vi "Main.vi"() -> ()   [LabVIEW 2010]
uses:
  <vilib>/Utility/config.llb/Read Key (Path).vi
  <vilib>/Utility/config.llb/Write Key (Path).vi
  DLL-s/MakeFullImmitationStepDLL/Release/MakeFullImmitationStepDLL.dll
  <vilib>/Utility/config.llb/NI_LVConfig.lvlib
panel:
  out "toChanger":T1(array[cluster])
  out "subpanel VI ref":refnum<vi>
  out "VP 2 GUI Msg Cluster Array":cluster{"Names":string[], "Codes":i32[]}
  out "selected path":path
  out "End Number":i32
  out "Project":string
  out "VP input vars":T2
  out "VP output vars":T3
  out "VM input vars":T2
  out "VM2SCM Msg Cluster Array":cluster{"Names":string[], "Codes":i32[]}
  out "VM INP from SCM Msg Cluster Array":cluster{"Names":string[], "Codes":i32[]}
  out "SCM2CA Msg Cluster Array":cluster{"Names":string[], "Codes":i32[]}
  out "SCM-SCM2VP Msg Cluster Array":cluster{"Names":string[], "Codes":i32[]}
  out "SCM2VM Msg Cluster Array":cluster{"Names":string[], "Codes":i32[]}
  out "VM2GUI Msg Cluster Array":cluster{"Names":string[], "Codes":i32[]}
  out "SCM STATES":string[][](array[string])
  out "SCM PROCESSES":string[](array[string])=["Инициализация", "ОстановВсехПроцессовИстартПроцИнициализация", "КонтрольДостоверности", "КонтрольДостоверностиОткрытияЗатвораВакуумного", "КонтрольДостоверностиОткрЗатВакуумного", "КонтрольДостоверностиЗакрЗатВакуумного", "КонтрольДостоверностиСостоянияСапуна", "КонтрольДостоверностиСостоянияУстройстваПлавПуска", "КонтрольДостоверностиСостоянияПитанияВакуумногоНасоса", "КонтрольДостоверностиСостоянияПитанияВентилятора", "КонтрольДостоверностиСостоянияПитанияРегТемпературы", "КонтрольДостоверностиСостоянияПитанияРегУровня", "КонтрольДостоверностиУровняВодыМинимум", "КонтрольДостоверностиУровняВодыМаксимум", "КонтрольДостоверностиСостоянияПитанияНасОхлаждения", "ЧтениеФактПараметров_с_Датчиков", "РЕГУЛЯТОР_ТРАФИКА", "ЧтениеКольцевогоБуфера", "ОбработкаКомандИзмененияНП_от_ГУИ", "ОбработкаКомандУправления_от_ГУИ", "КонтрольИзменения_ФП_P_ВбакеКомпрессора", "КонтрольИзменения_ФП_P_Впатрубке", "КонтрольИзменения_ФП_T_Врубашке", "КонтрольИзменения_ФП_T_Вбаке", "КонтрольИзменения_ФП_P_ВтрубеСидер", "КонтрольВеличиныОткачкиВауумнойТрубыСидеростата", "КонтрольГотовностиВакуума_в_Вакуумной_Трубе", "КонтрольУровняВодыБакаОхлаждения", "КонтрольТемпературыВодыБакаОхлаждения", "КонтрольТемпературыРубашкиОхлаждения", "КонтрольДавленияВбакеКомпрессора", "ВКЛ_ПИТ_ВЕНТИЛЯТОР", "ВЫК_ПИТ_ВЕНТИЛЯТОР", "КонтрольСостоянияПитанияВентилятора", "КонтрольСпонтанногоВыключенияВентилятора", "КонтрольСпонтанногоВключенияВентилятора", "КонтрольСостоянияЗатвораВакуумного", "ОТКР_ЗАТВОР_ВАК", "ЗАКР_ЗАТВОР_ВАК", "КонтрольСпонтанногоЗакрытияЗатвораВакуумного", "КонтрольСпонтанногоОткрытияЗатвораВакуумного", "ОТКР_САПУН", "ЗАКР_САПУН", "КонтрольСостоянияПитанияСапуна", "КонтрольСпонтанногоЗакрытияСапуна", "КонтрольСпонтанногоОткрытияСапуна", "ВКЛ_ПИТ_ВАК_НАСОСА", "ВЫК_ПИТ_ВАК_НАСОСА", "КонтрольСостоянияПитанияВакуумногоНасоса", "КонтрольСпонтанногоВыключенияВакНасоса", "КонтрольСпонтанногоВключенияВакНасоса", "ВКЛ_ПИТ_РЕГ_Т", "ВЫК_ПИТ_РЕГ_Т", "КонтрольСостоянияПитанияРЕГ_Т", "КонтрольСпонтанногоВыключенияРЕГ_Т", "КонтрольСпонтанногоВключенияРЕГ_Т", "ВКЛ_ПИТ_РЕГ_УР", "ВЫК_ПИТ_РЕГ_УР", "КонтрольСостоянияПитанияРЕГ_УР", "КонтрольСпонтанногоВыключенияРЕГ_УР", "КонтрольСпонтанногоВключенияРЕГ_УР", "ВКЛ_ПИТ_НАС_ОХЛ", "ВЫК_ПИТ_НАС_ОХЛ", "КонтрольСостоянияПитанияНАС_ОХЛ", "КонтрольСпонтанногоВыключенияНасосаОхлаждения", "КонтрольСпонтанногоВключенияНасосаОхлаждения", "ВКЛ_УСТР_ПЛАВ_ПУСКА", "ВЫК_УСТР_ПЛАВ_ПУСКА", "КонтрольСостоянияПитанияПЛАВ_ПУСКА", "КонтрольСпонтанногоВыключенияПлавнПуска", "КонтрольСпонтанногоВключенияПлавнПуска", "ВКЛ_ВАКУУМИРОВАНИЕ_ТРУБЫ", "ВЫК_ВАКУУМИРОВАНИЕ_ТРУБЫ", "ВКЛ_ВАКУУМНУЮ_ПОДСИСТЕМУ", "ВЫК_ВАКУУМНУЮ_ПОДСИСТЕМУ"]
  out "VM STATES":string[][](array[string])
  out "VM PROCESSES":string[](array[string])=["Инициализация", "ОстановВсехПроцессовИстартПроцИнициализация", "КонтрольДостоверности", "КонтрольДостоверностиОткрытияЗатвораВакуумного", "КонтрольДостоверностиОткрЗатВакуумного", "КонтрольДостоверностиЗакрЗатВакуумного", "КонтрольДостоверностиСостоянияСапуна", "КонтрольДостоверностиСостоянияУстройстваПлавПуска", "КонтрольДостоверностиСостоянияПитанияВакуумногоНасоса", "КонтрольДостоверностиСостоянияПитанияВентилятора", "КонтрольДостоверностиСостоянияПитанияРегТемпературы", "КонтрольДостоверностиСостоянияПитанияРегУровня", "КонтрольДостоверностиУровняВодыМинимум", "КонтрольДостоверностиУровняВодыМаксимум", "КонтрольДостоверностиСостоянияПитанияНасОхлаждения", "ЧтениеФактПараметров_с_Датчиков", "РЕГУЛЯТОР_ТРАФИКА", "ЧтениеКольцевогоБуфера", "ОбработкаКомандИзмененияНП_от_ГУИ", "ОбработкаКомандУправления_от_ГУИ", "КонтрольИзменения_ФП_P_ВбакеКомпрессора", "КонтрольИзменения_ФП_P_Впатрубке", "КонтрольИзменения_ФП_T_Врубашке", "КонтрольИзменения_ФП_T_Вбаке", "КонтрольИзменения_ФП_P_ВтрубеСидер", "КонтрольВеличиныОткачкиВауумнойТрубыСидеростата", "КонтрольГотовностиВакуума_в_Вакуумной_Трубе", "КонтрольУровняВодыБакаОхлаждения", "КонтрольТемпературыВодыБакаОхлаждения", "КонтрольТемпературыРубашкиОхлаждения", "КонтрольДавленияВбакеКомпрессора", "ВКЛ_ПИТ_ВЕНТИЛЯТОР", "ВЫК_ПИТ_ВЕНТИЛЯТОР", "КонтрольСостоянияПитанияВентилятора", "КонтрольСпонтанногоВыключенияВентилятора", "КонтрольСпонтанногоВключенияВентилятора", "КонтрольСостоянияЗатвораВакуумного", "ОТКР_ЗАТВОР_ВАК", "ЗАКР_ЗАТВОР_ВАК", "КонтрольСпонтанногоЗакрытияЗатвораВакуумного", "КонтрольСпонтанногоОткрытияЗатвораВакуумного", "ОТКР_САПУН", "ЗАКР_САПУН", "КонтрольСостоянияПитанияСапуна", "КонтрольСпонтанногоЗакрытияСапуна", "КонтрольСпонтанногоОткрытияСапуна", "ВКЛ_ПИТ_ВАК_НАСОСА", "ВЫК_ПИТ_ВАК_НАСОСА", "КонтрольСостоянияПитанияВакуумногоНасоса", "КонтрольСпонтанногоВыключенияВакНасоса", "КонтрольСпонтанногоВключенияВакНасоса", "ВКЛ_ПИТ_РЕГ_Т", "ВЫК_ПИТ_РЕГ_Т", "КонтрольСостоянияПитанияРЕГ_Т", "КонтрольСпонтанногоВыключенияРЕГ_Т", "КонтрольСпонтанногоВключенияРЕГ_Т", "ВКЛ_ПИТ_РЕГ_УР", "ВЫК_ПИТ_РЕГ_УР", "КонтрольСостоянияПитанияРЕГ_УР", "КонтрольСпонтанногоВыключенияРЕГ_УР", "КонтрольСпонтанногоВключенияРЕГ_УР", "ВКЛ_ПИТ_НАС_ОХЛ", "ВЫК_ПИТ_НАС_ОХЛ", "КонтрольСостоянияПитанияНАС_ОХЛ", "КонтрольСпонтанногоВыключенияНасосаОхлаждения", "КонтрольСпонтанногоВключенияНасосаОхлаждения", "ВКЛ_УСТР_ПЛАВ_ПУСКА", "ВЫК_УСТР_ПЛАВ_ПУСКА", "КонтрольСостоянияПитанияПЛАВ_ПУСКА", "КонтрольСпонтанногоВыключенияПлавнПуска", "КонтрольСпонтанногоВключенияПлавнПуска", "ВКЛ_ВАКУУМИРОВАНИЕ_ТРУБЫ", "ВЫК_ВАКУУМИРОВАНИЕ_ТРУБЫ", "ВКЛ_ВАКУУМНУЮ_ПОДСИСТЕМУ", "ВЫК_ВАКУУМНУЮ_ПОДСИСТЕМУ"]
  out "VP STATES":string[][](array[string])
  out "VP PROCESSES":string[](array[string])=["Инициализация", "ОстановВсехПроцессовИстартПроцИнициализация", "КонтрольДостоверности", "КонтрольДостоверностиОткрытияЗатвораВакуумного", "КонтрольДостоверностиОткрЗатВакуумного", "КонтрольДостоверностиЗакрЗатВакуумного", "КонтрольДостоверностиСостоянияСапуна", "КонтрольДостоверностиСостоянияУстройстваПлавПуска", "КонтрольДостоверностиСостоянияПитанияВакуумногоНасоса", "КонтрольДостоверностиСостоянияПитанияВентилятора", "КонтрольДостоверностиСостоянияПитанияРегТемпературы", "КонтрольДостоверностиСостоянияПитанияРегУровня", "КонтрольДостоверностиУровняВодыМинимум", "КонтрольДостоверностиУровняВодыМаксимум", "КонтрольДостоверностиСостоянияПитанияНасОхлаждения", "ЧтениеФактПараметров_с_Датчиков", "РЕГУЛЯТОР_ТРАФИКА", "ЧтениеКольцевогоБуфера", "ОбработкаКомандИзмененияНП_от_ГУИ", "ОбработкаКомандУправления_от_ГУИ", "КонтрольИзменения_ФП_P_ВбакеКомпрессора", "КонтрольИзменения_ФП_P_Впатрубке", "КонтрольИзменения_ФП_T_Врубашке", "КонтрольИзменения_ФП_T_Вбаке", "КонтрольИзменения_ФП_P_ВтрубеСидер", "КонтрольВеличиныОткачкиВауумнойТрубыСидеростата", "КонтрольГотовностиВакуума_в_Вакуумной_Трубе", "КонтрольУровняВодыБакаОхлаждения", "КонтрольТемпературыВодыБакаОхлаждения", "КонтрольТемпературыРубашкиОхлаждения", "КонтрольДавленияВбакеКомпрессора", "ВКЛ_ПИТ_ВЕНТИЛЯТОР", "ВЫК_ПИТ_ВЕНТИЛЯТОР", "КонтрольСостоянияПитанияВентилятора", "КонтрольСпонтанногоВыключенияВентилятора", "КонтрольСпонтанногоВключенияВентилятора", "КонтрольСостоянияЗатвораВакуумного", "ОТКР_ЗАТВОР_ВАК", "ЗАКР_ЗАТВОР_ВАК", "КонтрольСпонтанногоЗакрытияЗатвораВакуумного", "КонтрольСпонтанногоОткрытияЗатвораВакуумного", "ОТКР_САПУН", "ЗАКР_САПУН", "КонтрольСостоянияПитанияСапуна", "КонтрольСпонтанногоЗакрытияСапуна", "КонтрольСпонтанногоОткрытияСапуна", "ВКЛ_ПИТ_ВАК_НАСОСА", "ВЫК_ПИТ_ВАК_НАСОСА", "КонтрольСостоянияПитанияВакуумногоНасоса", "КонтрольСпонтанногоВыключенияВакНасоса", "КонтрольСпонтанногоВключенияВакНасоса", "ВКЛ_ПИТ_РЕГ_Т", "ВЫК_ПИТ_РЕГ_Т", "КонтрольСостоянияПитанияРЕГ_Т", "КонтрольСпонтанногоВыключенияРЕГ_Т", "КонтрольСпонтанногоВключенияРЕГ_Т", "ВКЛ_ПИТ_РЕГ_УР", "ВЫК_ПИТ_РЕГ_УР", "КонтрольСостоянияПитанияРЕГ_УР", "КонтрольСпонтанногоВыключенияРЕГ_УР", "КонтрольСпонтанногоВключенияРЕГ_УР", "ВКЛ_ПИТ_НАС_ОХЛ", "ВЫК_ПИТ_НАС_ОХЛ", "КонтрольСостоянияПитанияНАС_ОХЛ", "КонтрольСпонтанногоВыключенияНасосаОхлаждения", "КонтрольСпонтанногоВключенияНасосаОхлаждения", "ВКЛ_УСТР_ПЛАВ_ПУСКА", "ВЫК_УСТР_ПЛАВ_ПУСКА", "КонтрольСостоянияПитанияПЛАВ_ПУСКА", "КонтрольСпонтанногоВыключенияПлавнПуска", "КонтрольСпонтанногоВключенияПлавнПуска", "ВКЛ_ВАКУУМИРОВАНИЕ_ТРУБЫ", "ВЫК_ВАКУУМИРОВАНИЕ_ТРУБЫ", "ВКЛ_ВАКУУМНУЮ_ПОДСИСТЕМУ", "ВЫК_ВАКУУМНУЮ_ПОДСИСТЕМУ"]
  out "VP Cluster":T4
  out "CA output vars":T3
  out "CA input vars":T2
  out "CA2GUI Msg Cluster Array":cluster{"Names":string[], "Codes":i32[]}
  out "COM2CA MSG Cluster Array":cluster{"Names":string[], "Codes":i32[]}
  out "CA STATES":string[][](array[string])
  out "CA PROCESSES":string[](array[string])=["Инициализация", "ОстановВсехПроцессовИстартПроцИнициализация", "КонтрольДостоверности", "КонтрольДостоверностиОткрытияЗатвораВакуумного", "КонтрольДостоверностиОткрЗатВакуумного", "КонтрольДостоверностиЗакрЗатВакуумного", "КонтрольДостоверностиСостоянияСапуна", "КонтрольДостоверностиСостоянияУстройстваПлавПуска", "КонтрольДостоверностиСостоянияПитанияВакуумногоНасоса", "КонтрольДостоверностиСостоянияПитанияВентилятора", "КонтрольДостоверностиСостоянияПитанияРегТемпературы", "КонтрольДостоверностиСостоянияПитанияРегУровня", "КонтрольДостоверностиУровняВодыМинимум", "КонтрольДостоверностиУровняВодыМаксимум", "КонтрольДостоверностиСостоянияПитанияНасОхлаждения", "ЧтениеФактПараметров_с_Датчиков", "РЕГУЛЯТОР_ТРАФИКА", "ЧтениеКольцевогоБуфера", "ОбработкаКомандИзмененияНП_от_ГУИ", "ОбработкаКомандУправления_от_ГУИ", "КонтрольИзменения_ФП_P_ВбакеКомпрессора", "КонтрольИзменения_ФП_P_Впатрубке", "КонтрольИзменения_ФП_T_Врубашке", "КонтрольИзменения_ФП_T_Вбаке", "КонтрольИзменения_ФП_P_ВтрубеСидер", "КонтрольВеличиныОткачкиВауумнойТрубыСидеростата", "КонтрольГотовностиВакуума_в_Вакуумной_Трубе", "КонтрольУровняВодыБакаОхлаждения", "КонтрольТемпературыВодыБакаОхлаждения", "КонтрольТемпературыРубашкиОхлаждения", "КонтрольДавленияВбакеКомпрессора", "ВКЛ_ПИТ_ВЕНТИЛЯТОР", "ВЫК_ПИТ_ВЕНТИЛЯТОР", "КонтрольСостоянияПитанияВентилятора", "КонтрольСпонтанногоВыключенияВентилятора", "КонтрольСпонтанногоВключенияВентилятора", "КонтрольСостоянияЗатвораВакуумного", "ОТКР_ЗАТВОР_ВАК", "ЗАКР_ЗАТВОР_ВАК", "КонтрольСпонтанногоЗакрытияЗатвораВакуумного", "КонтрольСпонтанногоОткрытияЗатвораВакуумного", "ОТКР_САПУН", "ЗАКР_САПУН", "КонтрольСостоянияПитанияСапуна", "КонтрольСпонтанногоЗакрытияСапуна", "КонтрольСпонтанногоОткрытияСапуна", "ВКЛ_ПИТ_ВАК_НАСОСА", "ВЫК_ПИТ_ВАК_НАСОСА", "КонтрольСостоянияПитанияВакуумногоНасоса", "КонтрольСпонтанногоВыключенияВакНасоса", "КонтрольСпонтанногоВключенияВакНасоса", "ВКЛ_ПИТ_РЕГ_Т", "ВЫК_ПИТ_РЕГ_Т", "КонтрольСостоянияПитанияРЕГ_Т", "КонтрольСпонтанногоВыключенияРЕГ_Т", "КонтрольСпонтанногоВключенияРЕГ_Т", "ВКЛ_ПИТ_РЕГ_УР", "ВЫК_ПИТ_РЕГ_УР", "КонтрольСостоянияПитанияРЕГ_УР", "КонтрольСпонтанногоВыключенияРЕГ_УР", "КонтрольСпонтанногоВключенияРЕГ_УР", "ВКЛ_ПИТ_НАС_ОХЛ", "ВЫК_ПИТ_НАС_ОХЛ", "КонтрольСостоянияПитанияНАС_ОХЛ", "КонтрольСпонтанногоВыключенияНасосаОхлаждения", "КонтрольСпонтанногоВключенияНасосаОхлаждения", "ВКЛ_УСТР_ПЛАВ_ПУСКА", "ВЫК_УСТР_ПЛАВ_ПУСКА", "КонтрольСостоянияПитанияПЛАВ_ПУСКА", "КонтрольСпонтанногоВыключенияПлавнПуска", "КонтрольСпонтанногоВключенияПлавнПуска", "ВКЛ_ВАКУУМИРОВАНИЕ_ТРУБЫ", "ВЫК_ВАКУУМИРОВАНИЕ_ТРУБЫ", "ВКЛ_ВАКУУМНУЮ_ПОДСИСТЕМУ", "ВЫК_ВАКУУМНУЮ_ПОДСИСТЕМУ"]
  out "CA DESCR":T5
  out "VM DESCR":T6
  out "exists":bool
  out "Scalar":bool
  in  "Проект":path
  out "Stop Ver Button":bool
  in  "Pause":bool
  out "Верификация запущена":bool
  out "error":i32
  in  "verifier2scenariousControlOutMsgs":cluster{"MSG":i16, "param":i32, "Type":i16}[](array[cluster])
  out "Verification":bool
  in  "scenarioStates":cluster{"TimeInState":u16, "cur_state":i8}[](array[cluster])
  in  "verStates":cluster{"TimeInState":u16, "cur_state":i8}[](array[cluster])
  in  "vplantStates":cluster{"TimeInState":u16, "cur_state":i8}[](array[cluster])
  in  "algStates":cluster{"TimeInState":u16, "cur_state":i8}[](array[cluster])
  in  "virtualPlant2GUIOutputMsgs":cluster{"MSG":i16, "param":i32, "Type":i16}[](array[cluster])
  in  "verifier2GUIOutputMsgs":cluster{"MSG":i16, "param":i32, "Type":i16}[](array[cluster])
  in  "algOutputMsgs":T7(array[cluster])
  in  "scenarios2VerifierOutputMsgs":cluster{"MSG":i16, "param":i32, "Type":i16}[](array[cluster])
  in  "scenarios2VirtPlantOutputMsgs":cluster{"MSG":i16, "param":i32, "Type":i16}[](array[cluster])
  in  "scenarios2AlgOutputMsgs":cluster{"MSG":i16, "param":i32, "Type":i16}[](array[cluster])
  in  "algOutputPorts":i8[](array[numeric])
  in  "algInputPorts":i8[](array[numeric])
  in  "TEST MODE":bool
  in  "Open editor":bool
  in  "START Button":bool
  out "VM vi reference":refnum<vi> caption="CA vi reference"
  out "SCB vi reference":refnum<vi> caption="CA vi reference"
  out "VP vi reference":refnum<vi> caption="CA vi reference"
  out "CA vi reference":refnum<vi>
  out "error out":errorcluster
  in  "Открыть панель БВ":bool
  in  "Открыть панель БУС":bool
  in  "Открыть панель АУ":bool
  in  "stop":bool
  in  "Открыть панель ВОУ":bool
  out "Автоматический режим работы":bool
  in  "Режим работы:":bool
  # "Ручной"
  # "Автоматический"
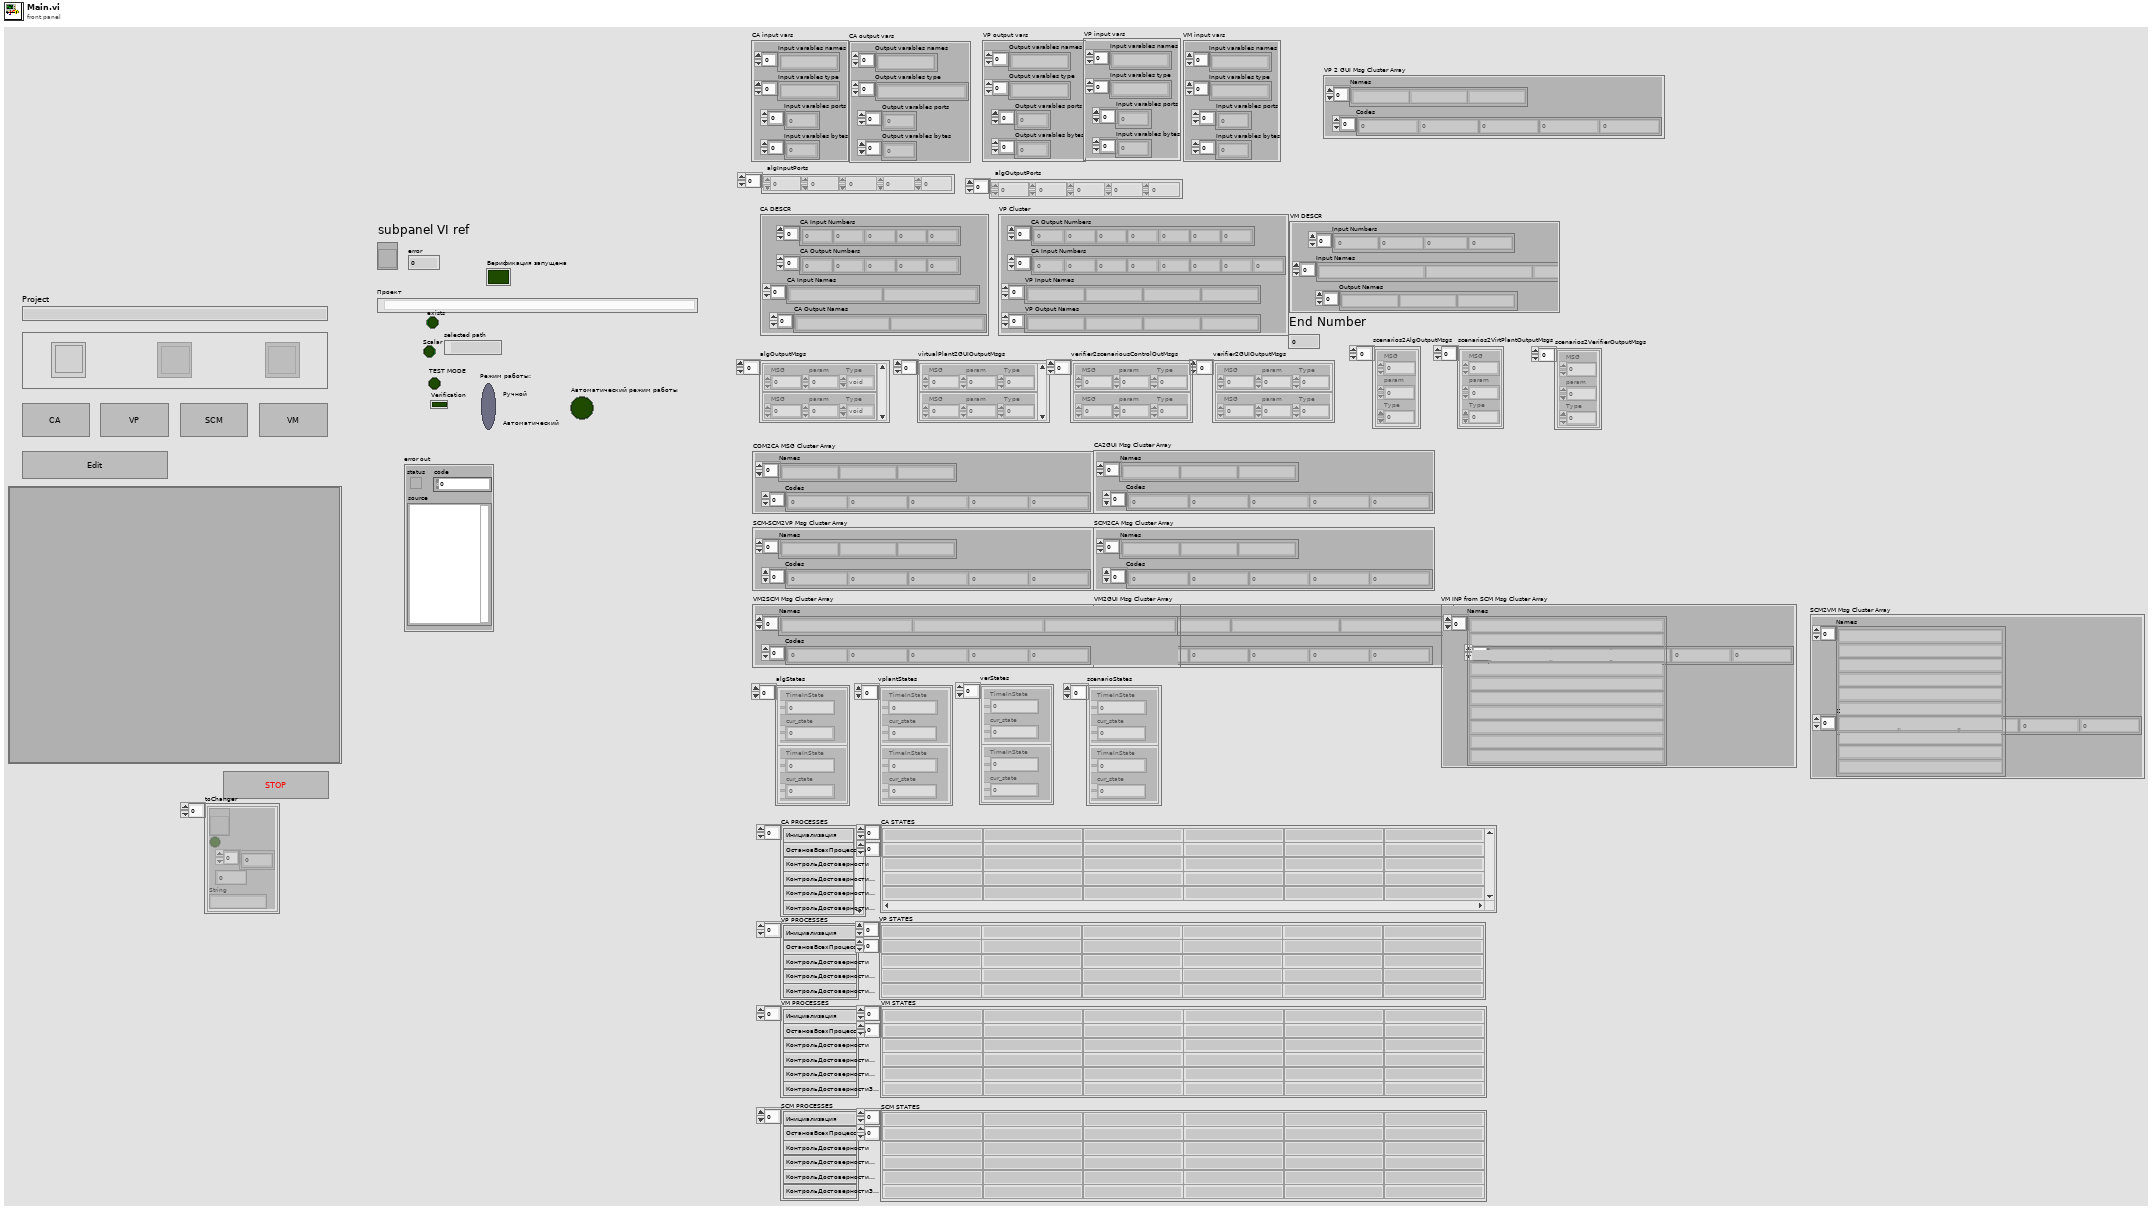
[diagram p1: front panel]
types:
  T1 = cluster{refnum<vi>, bool, i32[], i32, "String":string}[]
  T2 = cluster{"Input varables names":string[], "Input varables type":string[], "Input varables ports":i32[], "Input varables bytes":i32[]}
  T3 = cluster{"Output varables names":string[], "Output varables type":string[], "Output varables ports":i32[], "Output varables bytes":i32[]}
  T4 = cluster{"CA Output Numbers ":i32[], "CA Input Numbers":i32[], "VP Input Names":string[], "VP Output Names ":string[]}
  T5 = cluster{"CA Input Numbers":i32[], "CA Output Numbers ":i32[], "CA Input Names":string[], "CA Output Names ":string[]}
  T6 = cluster{"Input Numbers":i32[], "Input Names":string[], "Output Names ":string[]}
  T7 = cluster{"MSG":i16, "param":i32, "Type":enum16{"void", "byte", "int", "float"}}[]
  T8 = enum8{"Enabled", "Disabled", "Disabled and Grayed Out"}
  T9 = typedef "NI_LVConfig.lvlib/Config Data RefNum.ctl" = refnum<k1>
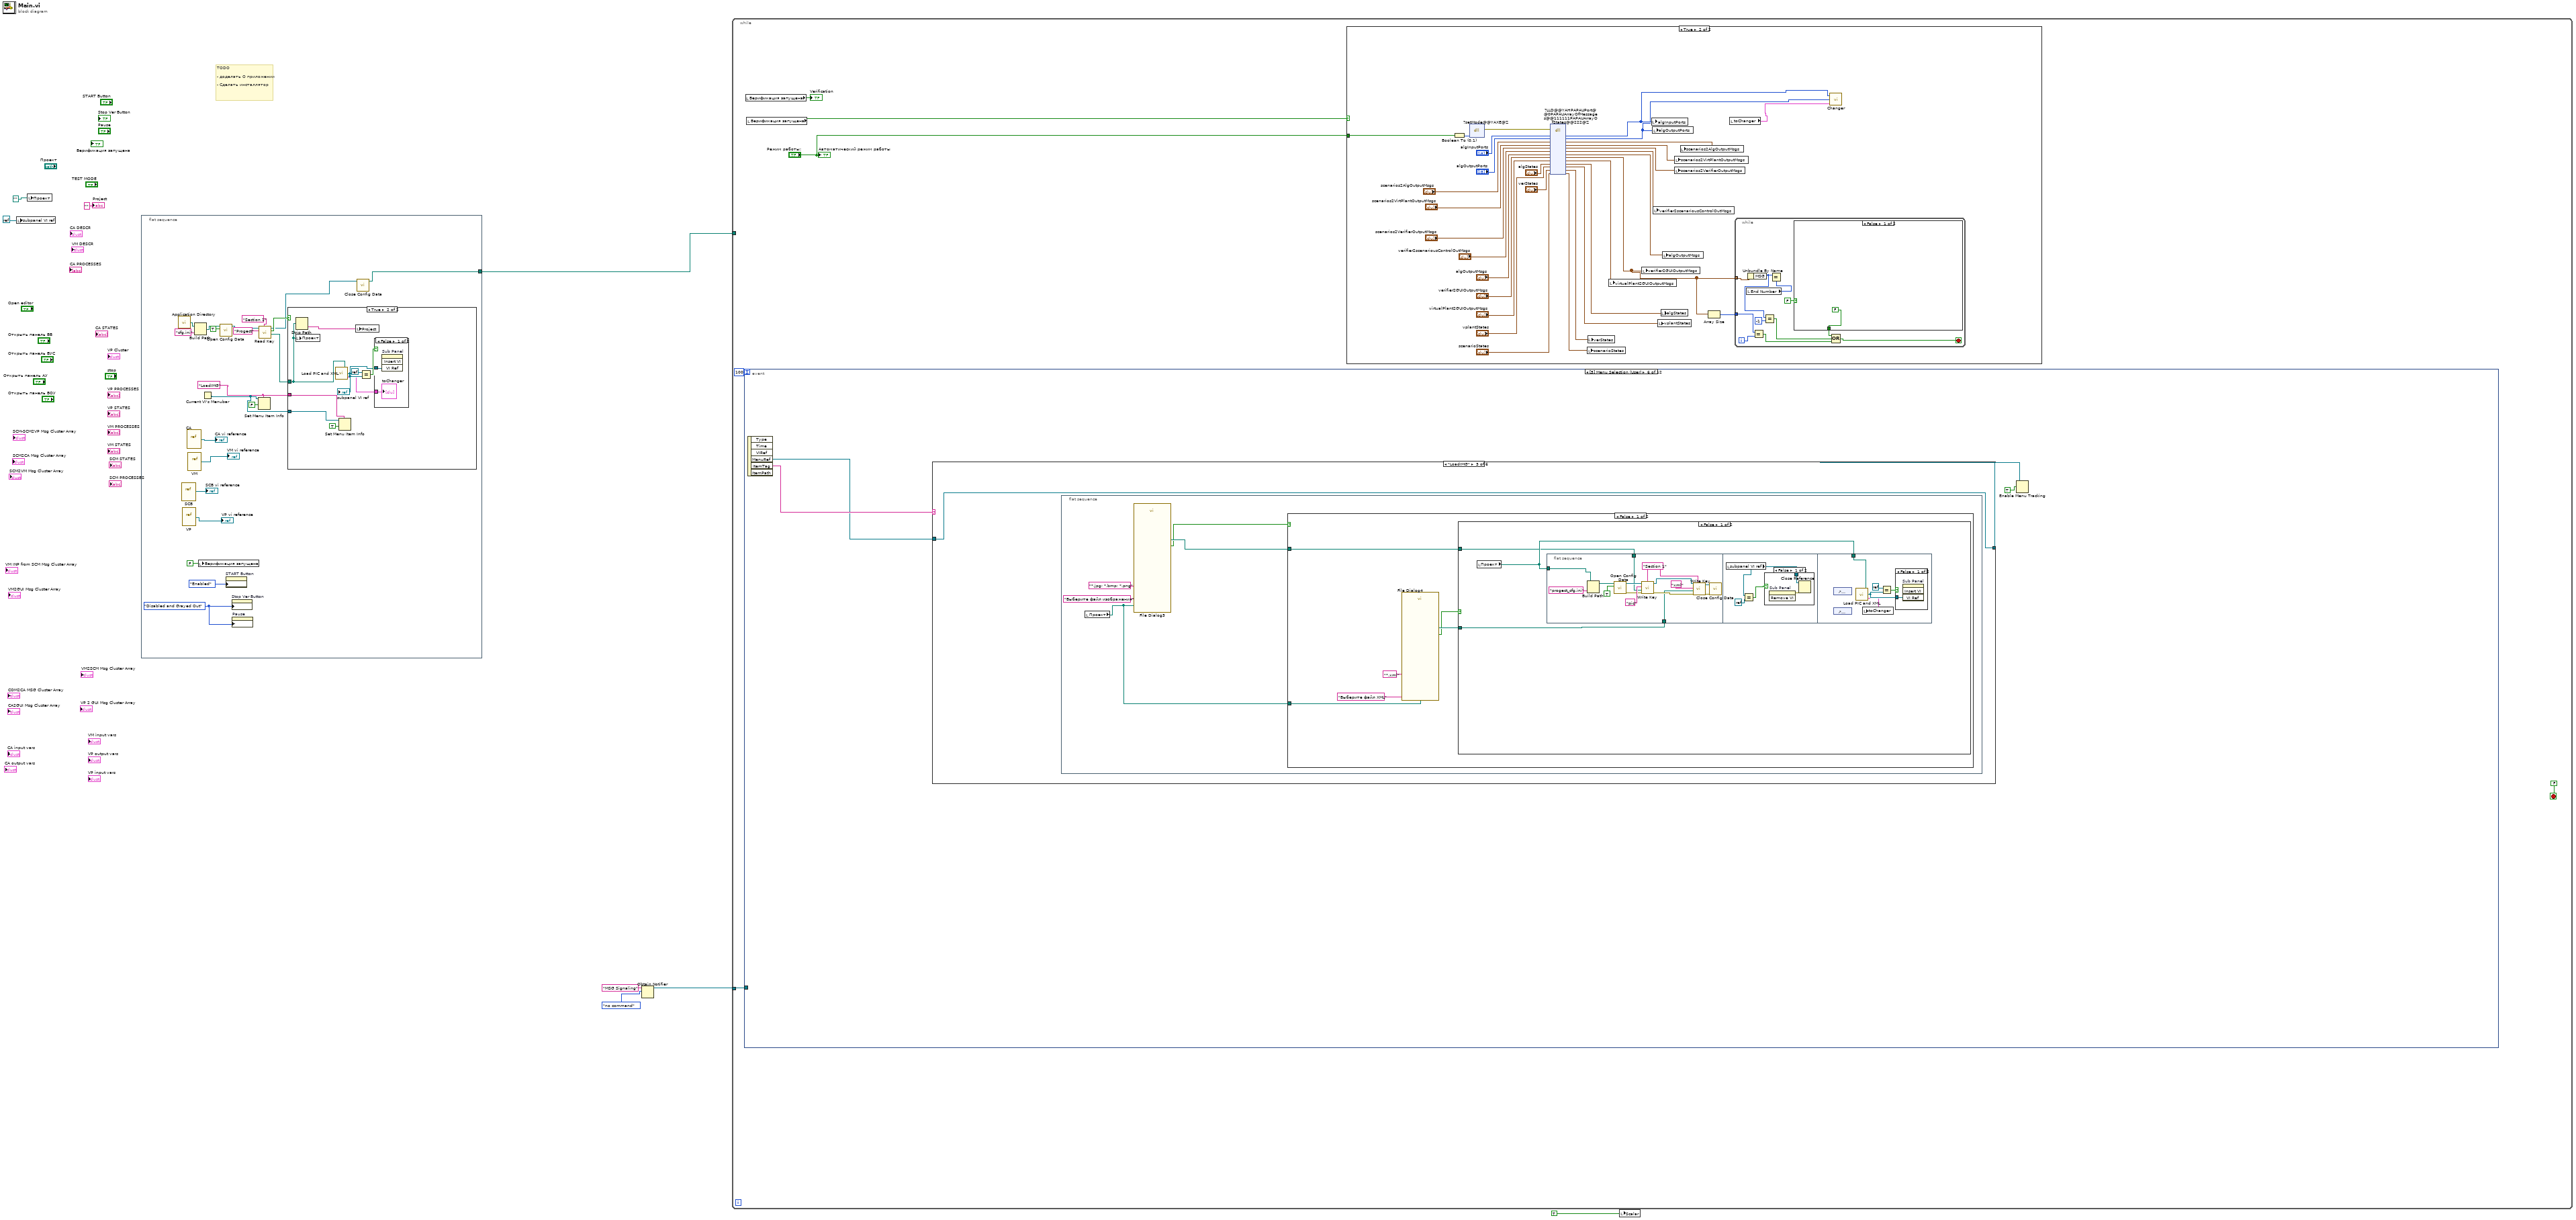
[diagram p0: block diagram]
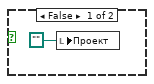
[diagram p2: hidden frame]
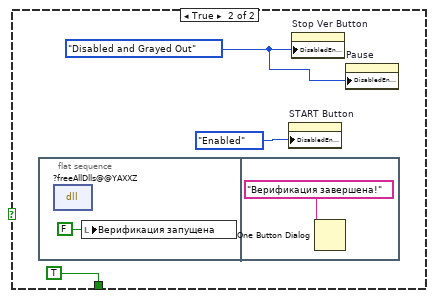
[diagram p5: hidden frame]
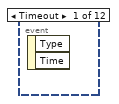
[diagram p6: hidden frame]
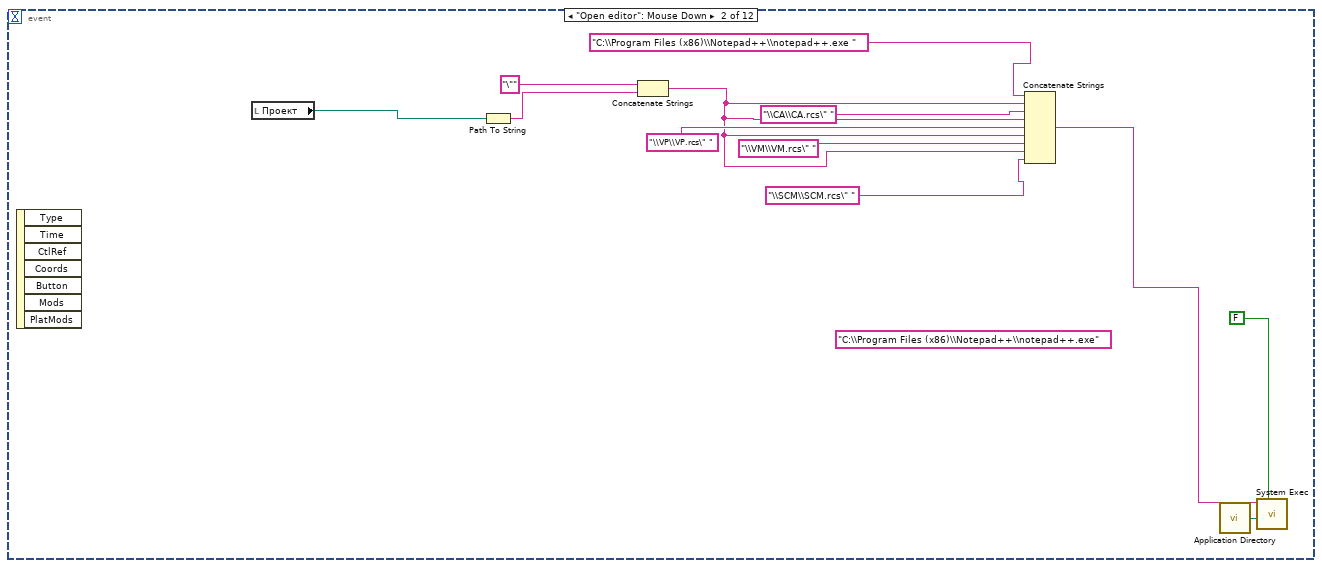
[diagram p7: hidden frame]
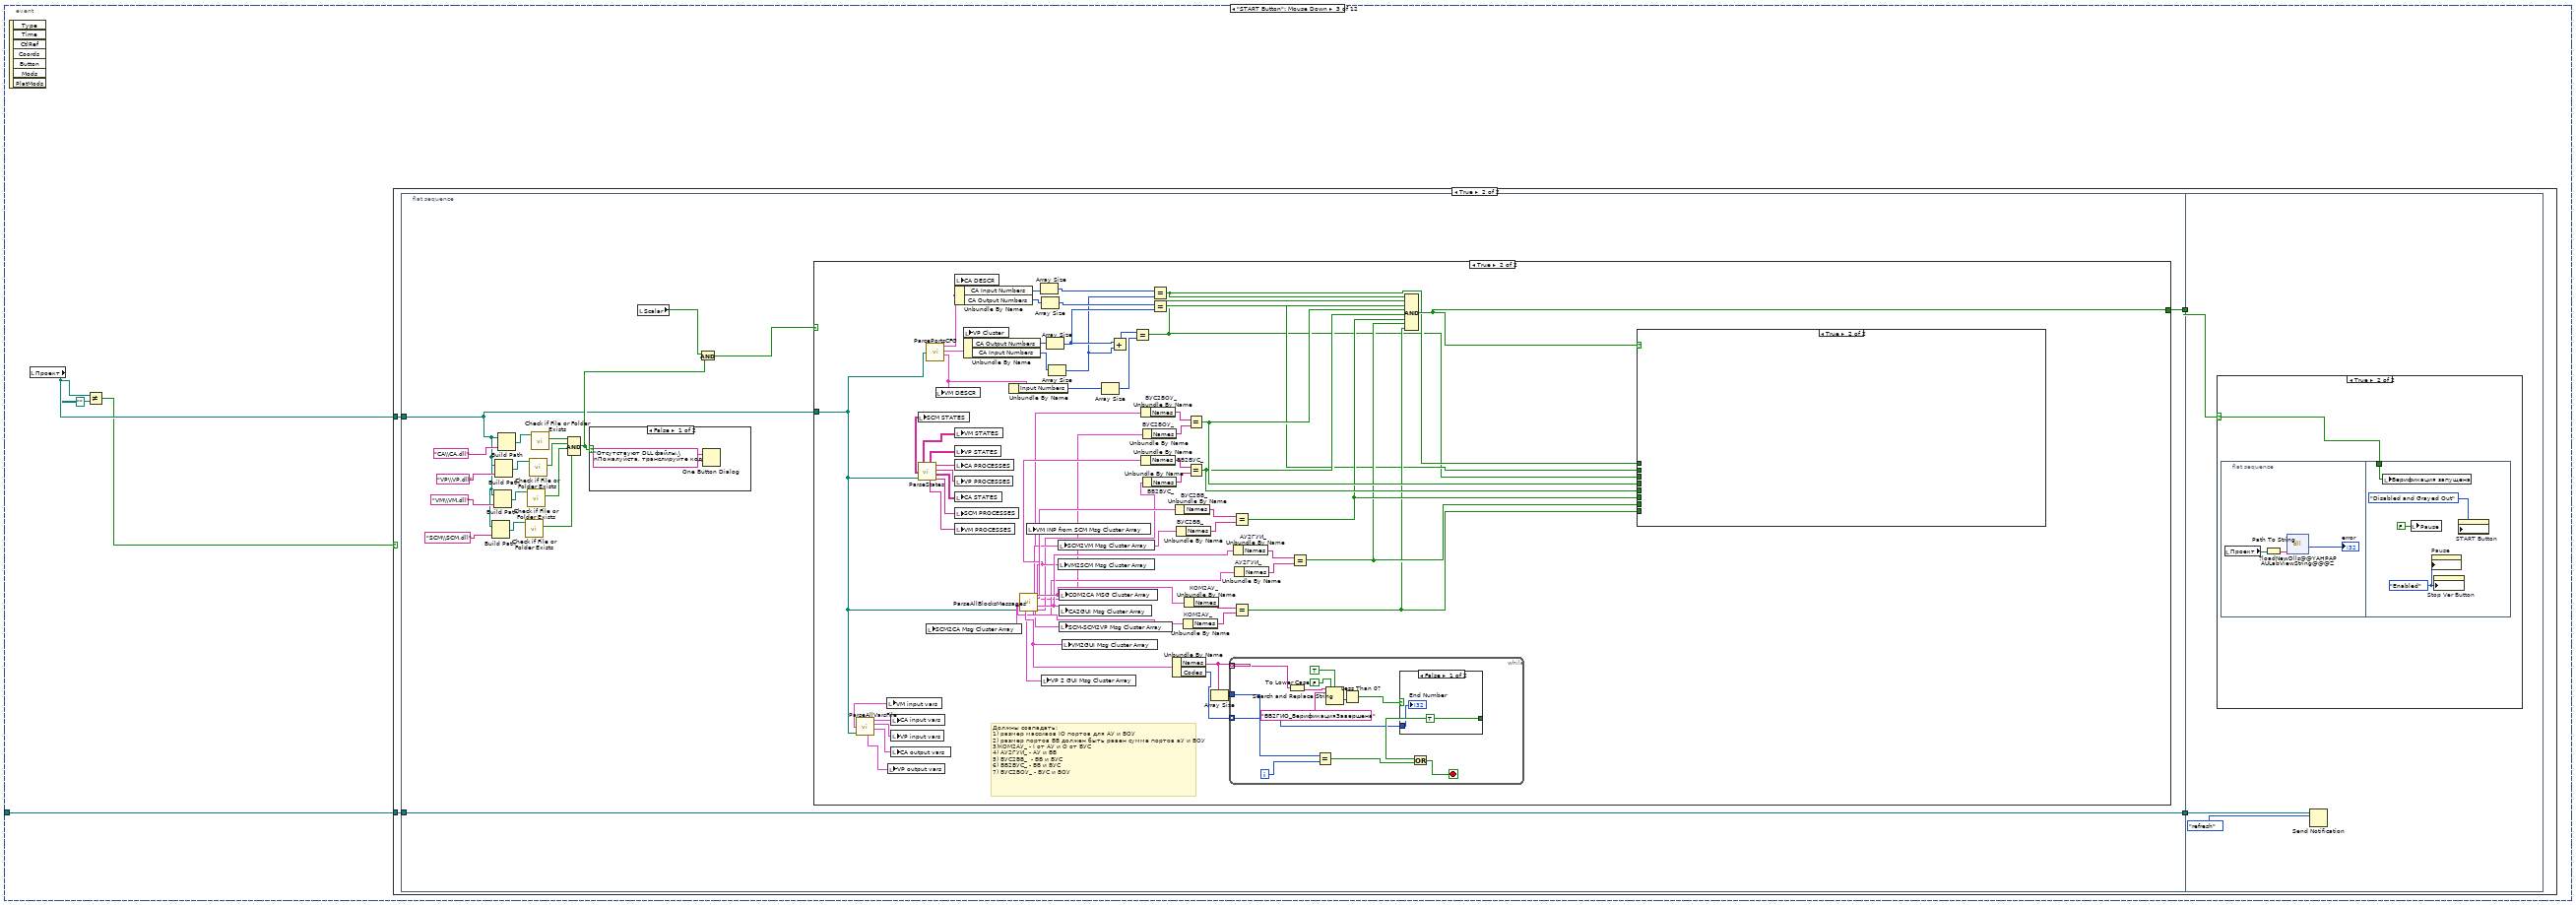
[diagram p8: hidden frame]
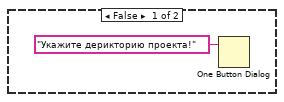
[diagram p9: hidden frame]
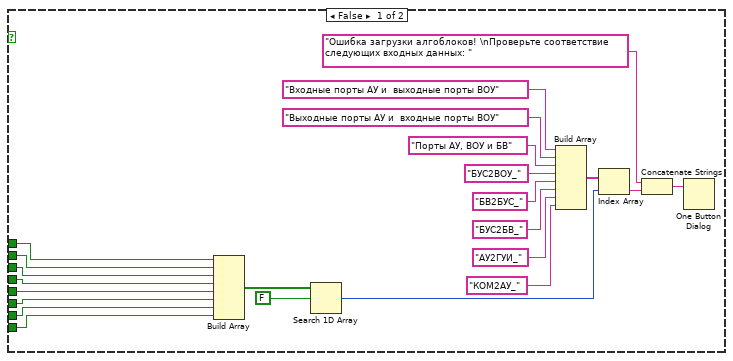
[diagram p12: hidden frame]
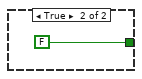
[diagram p13: hidden frame]
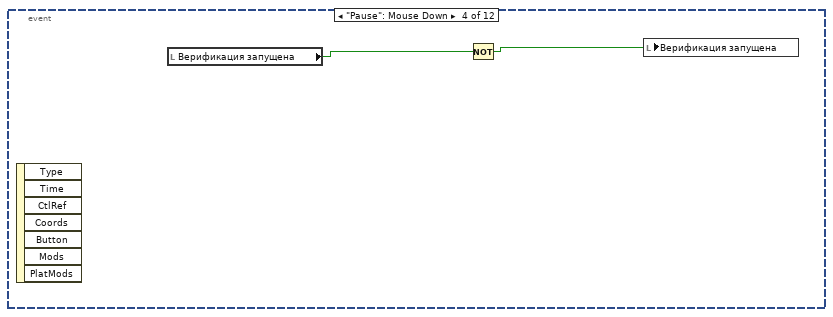
[diagram p15: hidden frame]
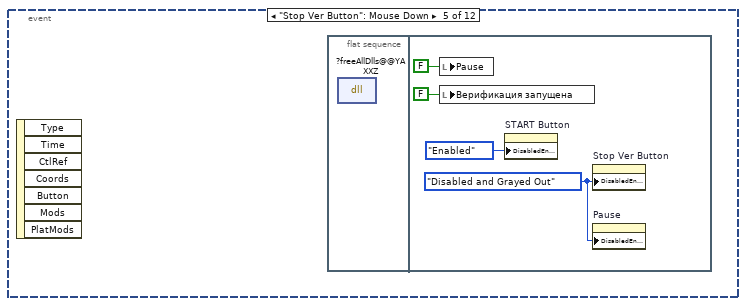
[diagram p16: hidden frame]
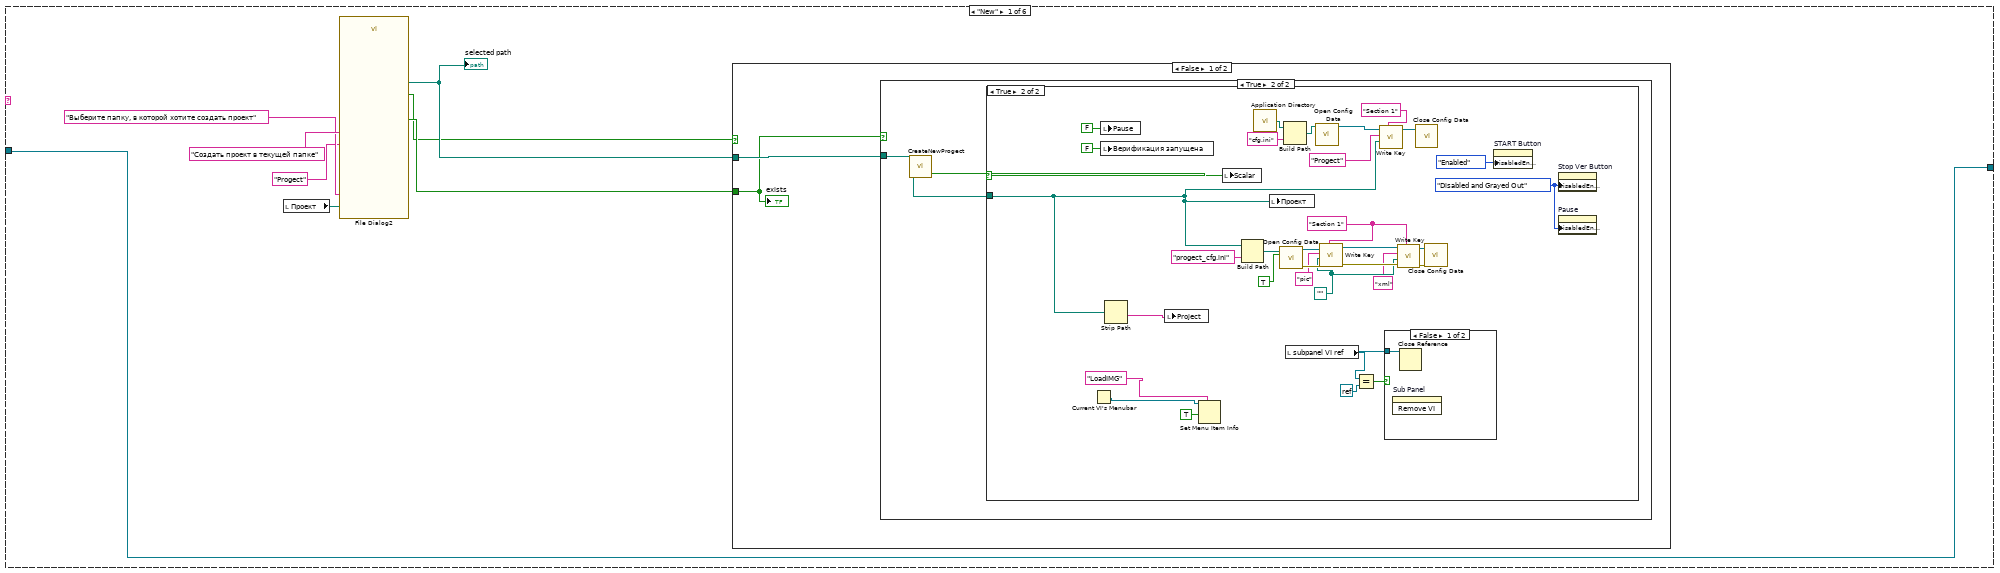
[diagram p17: hidden frame]
diagram:
  # "TODO\n\n- доделать О приложении\n\n- Сделать инсталлятор"
  n1 = local write "subpanel VI ref"(refnum<k0> refnum) -> ()
  n2 = local write "Проект"(path "") -> ()
  n3 = flat-sequence {
    tunnel: [w16] -> w3
    frame #0 {
      w14 = "LoadIMG" ("item tag")
      w27 = T8."Disabled and Grayed Out" ("Disabled")
      n4 = call <vilib>:"Application Directory.vi"() -> ("Application Directory"=w26:path)
      n5 = vi-ref "SCB.vi"() -> (→"SCB vi reference":refnum<vi>)
      n6 = vi-ref "VP.vi"() -> (→"VP vi reference":refnum<vi>)
      n7 = vi-ref "CA.vi"() -> (→"CA vi reference":refnum<vi>)
      n8 = vi-ref "VM.vi"() -> (→"VM vi reference":refnum<vi>)
      n9 = Build Path(base path=w26, name or relative path="cfg.ini") -> (appended path=w24:path)
      n10 = local write "Верификация запущена"(FALSE ("VerificationRunning")) -> ()
      n11 = Current VI's Menubar() -> (w13:refnum<k9>)
      n12 = call <vilib>:"Open Config Data.vi"("create file if necessary (T)"=TRUE, "configuration file path"=w24) -> ("refnum"=w19:T9)  [unwired: 7 in, 2 out]
      n13 = property on="START Button" class="Bool (strict)"("DisabledEnum"=T8."Enabled" ("Disabled")) -> ()  [unwired: 2 in, 2 out]
      n14 = property on="Stop Ver Button" class="Bool (strict)"("DisabledEnum"=w27) -> ()  [unwired: 2 in, 2 out]
      n15 = property on="Pause" class="Bool (strict)"("DisabledEnum"=w27) -> ()  [unwired: 2 in, 2 out]
      n16 = Set Menu Item Info(7:w14, 9:FALSE ("enabled"), 11:w13) -> ()  [unwired: 4 in, 2 out]
      n17 = call-poly <vilib>:"Read Key.vi"("section"="Section 1", "key"="Progect", "refnum"=w19) -> ("value"=w20:path, "found?"=w21:bool, "refnum out"=w17:T9)  [unwired: 5 in, 1 out]
      n18 = case shown="True" w21 {
        tunnel: w20 -> [_ w39]
        tunnel: w14 -> [_ w33]
        tunnel: w13 -> [_ w32]
        frame False {
          n19 = local write "Проект"(path "") -> ()
        }
        frame True {
          n20 = Strip Path(path=w39) -> (name=w35:string)  [unwired: 1 out]
          n21 = local write "Проект"(w39) -> ()
          n22 = call "Load PIC and XML.vi"("selected path"=w39) -> ("toChanger"=w31:T1, "vi refnum"=w36:refnum<vi>)  [unwired: 2 in]
          "subpanel VI ref" <- w36
          n23 = Set Menu Item Info(7:w33, 9:TRUE ("enabled"), 11:w32) -> ()  [unwired: 4 in, 2 out]
          n24 = local write "Project"(w35) -> ()
          n25 = Equal?(x=refnum<k0> refnum, y=w36) -> (x = y?=w37:bool)
          n26 = case shown="False" w37 {
            tunnel: w36 -> [w41 _]
            tunnel: w31 -> [w40 _]
            frame False {
              n27 = invoke on="Sub Panel" class="SubPnl" method="Insert VI"("VI Ref"=w41) -> ()  [unwired: 3 in, 4 out]
              "toChanger" <- w40
            }
            frame True {
            }
          }
        }
      }
      n28 = call <vilib>:"Close Config Data.vi"("refnum"=w17) -> ("file path"=w16:path)  [unwired: 9 in, 1 out]
    }
  }
  n29 = Obtain Notifier(name (unnamed)="MSG Signaling", notification data type=enum16{"no command", "refresh"}."no command") -> (notifier out=w6:refnum<notifier>)  [unwired: 2 in, 2 out]
  n30 = while {
    tunnel: w6 -> [w43]
    tunnel: w3 -> [_]
    stop <- FALSE ("stop") stop-if-true
    n31 = event shown="[5] Menu Selection (User)" {
      selector: _ -> [_ _ _ _ _ _ _ _ _ _ _ _]
      dyn-events: _ -> [_ _ _ _ _ _ _ _ _ _ _ _]
      timeout: 100 -> [_ _ _ _ _ _ _ _ _ _ _ _]
      tunnel: w43 -> [_ _ w111 _ _ _ _ _ _ _ _ _]
      event Timeout {
        n32 = event-data() -> ()  [unwired: 1 in, 2 out]
      }
      event "Open editor": Mouse Down {
        (unwired) "C:\\Program Files (x86)\\Notepad++\\notepad++.exe" ("command line")
        n33 = event-data() -> ()  [unwired: 1 in, 7 out]
        n34 = local read "Проект"() -> (w100:path)
        n35 = Path To String(path=w100) -> (string=w102:string)
        n36 = Concatenate Strings("\"" ("string"), w102) -> (w98:string)
        n37 = Concatenate Strings("C:\\Program Files (x86)\\Notepad++\\notepad++.exe " ("command line"), w98, "\\CA\\CA.rcs\" " ("string"), w98, "\\VP\\VP.rcs\" " ("string"), w98, "\\VM\\VM.rcs\" " ("string"), w98, "\\SCM\\SCM.rcs\" " ("string")) -> (w96:string)
        n38 = call <vilib>:"Application Directory.vi"() -> ("Application Directory"=w106:path)
        n39 = call <vilib>:"System Exec.vi"("wait until completion? (T)"=FALSE, "working directory"=w106, "command line"=w96) -> ()  [unwired: 5 in, 4 out]
      }
      event "START Button": Mouse Down {
        n40 = event-data() -> ()  [unwired: 1 in, 7 out]
        n41 = local read "Проект"() -> (w110:path)
        n42 = Not Equal?(x=w110, y=path "") -> (x != y?=w108:bool)
        n43 = case shown="True" w108 {
          tunnel: w111 -> [_ w114]
          tunnel: w110 -> [_ w113]
          frame False {
            n44 = One Button Dialog(message="Укажите дерикторию проекта!") -> ()  [unwired: 1 in, 1 out]
          }
          frame True {
            n45 = flat-sequence {
              tunnel: w114 -> [w134]
              tunnel: [w134] -> w116
              tunnel: [w133] -> w115
              tunnel: w113 -> [w117]
              tunnel: w116 -> [w240]
              tunnel: w115 -> [w238]
              frame #0 {
                n46 = Build Path(base path=w117, name or relative path="SCM\\SCM.dll") -> (appended path=w127:path)
                n47 = Build Path(base path=w117, name or relative path="VM\\VM.dll") -> (appended path=w128:path)
                n48 = Build Path(base path=w117, name or relative path="VP\\VP.dll") -> (appended path=w129:path)
                n49 = Build Path(base path=w117, name or relative path="CA\\CA.dll") -> (appended path=w131:path)
                n50 = call <vilib>:"Check if File or Folder Exists.vi"("path"=w127) -> ("file or folder exists?"=w118:bool)  [unwired: 8 in, 2 out]
                n51 = call <vilib>:"Check if File or Folder Exists.vi"("path"=w128) -> ("file or folder exists?"=w122:bool)  [unwired: 8 in, 2 out]
                n52 = call <vilib>:"Check if File or Folder Exists.vi"("path"=w129) -> ("file or folder exists?"=w123:bool)  [unwired: 8 in, 2 out]
                n53 = call <vilib>:"Check if File or Folder Exists.vi"("path"=w131) -> ("file or folder exists?"=w130:bool)  [unwired: 8 in, 2 out]
                n54 = Compound Arithmetic op=AND(w130, w123, w122, w118) -> (w121:bool)
                n55 = case shown="False" w121 {
                  frame False {
                    n56 = One Button Dialog(message="Отсутствуют DLL файлы.\nПожалуйста, транслируйте код.") -> ()  [unwired: 1 in, 1 out]
                  }
                  frame True {
                  }
                }
                n57 = local read "Scalar"() -> (w120:bool)
                n58 = And(x=w120, y=w121) -> (x .and. y?=w119:bool)
                n59 = case shown="True" w119 {
                  selector: w119 -> [w136 _]
                  tunnel: [w136 w142] -> w133
                  tunnel: w117 -> [_ w138]
                  frame False {
                  }
                  frame True {
                    # "Должны совпадать:\n1) размер массивов IO портов для АУ и ВОУ\n2) размер портов БВ должен быть равен сумме портов аУ и ВОУ\n3)КОМ2АУ_ - I от АУ и O от БУС\n4) АУ2ГУИ_ - АУ и БВ\n5) БУС2БВ_  - БВ и БУС\n6) БВ2БУС_ - БВ и БУС\n7) БУС2ВОУ_ - БУС и ВОУ"
                    n60 = call "ParseAllVarsFile.vi"("Path"=w138) -> ("CA input vars"=w196:T2, "VP input vars"=w186:T2, "CA output vars"=w195:T3, "VP output vars"=w187:T3, "VM input vars"=w188:T2)  [unwired: 3 out]
                    n61 = local write "VM input vars"(w188) -> ()
                    n62 = local write "VP output vars"(w187) -> ()
                    n63 = local write "CA input vars"(w196) -> ()
                    n64 = local write "VP input vars"(w186) -> ()
                    n65 = local write "CA output vars"(w195) -> ()
                    n66 = call "ParseStates.vi"("base path"=w138) -> ("CA PROCESSES"=w198:string[], "VP STATES"=w193:string[][], "VP PROCESSES"=w194:string[], "CA STATES"=w197:string[][], "VM PROCESSES"=w192:string[], "SCM PROCESSES"=w190:string[], "VM STATES"=w191:string[][], "SCM STATES"=w189:string[][])
                    n67 = local write "SCM STATES"(w189) -> ()
                    n68 = call "ParcePortsCFG.vi"("path"=w138) -> ("VM Cluster"=w174:T6, "VP Cluster"=w181:T4, "CA Cluster"=w182:T5)  [unwired: 1 out]
                    n69 = local write "VM DESCR"(w174) -> ()
                    n70 = local write "CA DESCR"(w182) -> ()
                    n71 = Unbundle By Name(w182) -> ("CA Input Numbers"=w180:i32[], "CA Output Numbers"=w179:i32[])
                    n72 = local write "VM STATES"(w191) -> ()
                    n73 = local write "VP STATES"(w193) -> ()
                    n74 = local write "CA PROCESSES"(w198) -> ()
                    n75 = local write "VP PROCESSES"(w194) -> ()
                    n76 = local write "CA STATES"(w197) -> ()
                    n77 = local write "SCM PROCESSES"(w190) -> ()
                    n78 = local write "VM PROCESSES"(w192) -> ()
                    n79 = local write "VP Cluster"(w181) -> ()
                    n80 = Unbundle By Name(w181) -> ("CA Output Numbers"=w178:i32[], "CA Input Numbers"=w177:i32[])
                    n81 = Unbundle By Name(w174) -> ("Input Numbers"=w173:i32[])
                    n82 = call "ParseAllBlocksMessages.vi"("Path"=w138) -> ("SCM2VM Msg Cluster Array"=w153:cluster{"Names":string[], "Codes":i32[]}, "VM INP from SCM Msg Cluster Array"=w157:cluster{"Names":string[], "Codes":i32[]}, "VM2SCM Msg Cluster Array"=w154:cluster{"Names":string[], "Codes":i32[]}, "COM2CA MSG Cluster Array"=w168:cluster{"Names":string[], "Codes":i32[]}, "SCM-SCM2VP Msg Cluster Array"=w149:cluster{"Names":string[], "Codes":i32[]}, "VP-SCM2VP Msg Cluster Array"=w148:cluster{"Names":string[], "Codes":i32[]}, "SCM2CA Msg Cluster Array"=w166:cluster{"Names":string[], "Codes":i32[]}, "CA2GUI Msg Cluster Array"=w163:cluster{"Names":string[], "Codes":i32[]}, "VM2GUI Msg Cluster Array"=w167:cluster{"Names":string[], "Codes":i32[]}, "VP 2 GUI Msg Cluster Array"=w137:cluster{"Names":string[], "Codes":i32[]}, "VM INP from CA Msg Cluster Array"=w162:cluster{"Names":string[], "Codes":i32[]}, "SCM - VM2SCM Msg Cluster Array"=w152:cluster{"Names":string[], "Codes":i32[]})  [unwired: 3 in]
                    n83 = local write "SCM2CA Msg Cluster Array"(w166) -> ()
                    n84 = local write "VM INP from SCM Msg Cluster Array"(w157) -> ()
                    n85 = Array Size(array=w180) -> (size(s)=w175:i32)
                    n86 = Array Size(array=w179) -> (size(s)=w176:i32)
                    n87 = local write "VP 2 GUI Msg Cluster Array"(w137) -> ()
                    n88 = Array Size(array=w178) -> (size(s)=w172:i32)
                    n89 = Array Size(array=w177) -> (size(s)=w171:i32)
                    n90 = local write "SCM2VM Msg Cluster Array"(w153) -> ()
                    n91 = local write "VM2SCM Msg Cluster Array"(w154) -> ()
                    n92 = local write "COM2CA MSG Cluster Array"(w168) -> ()
                    n93 = local write "CA2GUI Msg Cluster Array"(w163) -> ()
                    n94 = local write "SCM-SCM2VP Msg Cluster Array"(w149) -> ()
                    n95 = local write "VM2GUI Msg Cluster Array"(w167) -> ()
                    n96 = Array Size(array=w173) -> (size(s)=w169:i32)
                    n97 = Add(x=w172, y=w171) -> (x+y=w170:i32)
                    n98 = Equal?(x=w170, y=w169) -> (x = y?=w139:bool)
                    n99 = Unbundle By Name "БУС2ВОУ_"(w149) -> ("Names"=w150:string[])
                    n100 = Unbundle By Name "БВ2БУС_"(w154) -> ("Names"=w156:string[])
                    n101 = Unbundle By Name "БУС2ВОУ_"(w148) -> ("Names"=w151:string[])
                    n102 = Unbundle By Name "БВ2БУС_"(w152) -> ("Names"=w155:string[])
                    n103 = Equal?(x=w175, y=w171) -> (x = y?=w141:bool)
                    n104 = Equal?(x=w176, y=w172) -> (x = y?=w140:bool)
                    n105 = Unbundle By Name(w167) -> ("Names"=w185:string[], "Codes"=w183:i32[])
                    n106 = Unbundle By Name "БУС2БВ_"(w157) -> ("Names"=w159:string[])
                    n107 = Unbundle By Name "БУС2БВ_"(w153) -> ("Names"=w158:string[])
                    n108 = Unbundle By Name "КОМ2АУ_"(w166) -> ("Names"=w164:string[])
                    n109 = Unbundle By Name "КОМ2АУ_"(w168) -> ("Names"=w165:string[])
                    n110 = Equal?(x=w150, y=w151) -> (x = y?=w147:bool)
                    n111 = Equal?(x=w156, y=w155) -> (x = y?=w146:bool)
                    n112 = Array Size(array=w185) -> (size(s)=w184:i32)
                    n113 = while {
                      tunnel: w185 -> [w229] mode=indexing
                      tunnel: w184 -> [w226]
                      tunnel: w183 -> [w222] mode=indexing
                      i -> [w227]
                      stop <- w223 stop-if-true
                      n114 = To Lower Case(string=w229) -> (all lower case string=w228:string)
                      n115 = Equal?(x=w226, y=w227) -> (x = y?=w225:bool)
                      n116 = Search and Replace String(replace all?=FALSE ("replace all? (F)"), case sensitive?=TRUE ("ignore case? (F)"), input string=w228, search string="БВ2ГИО_ВерификацияЗавершена") -> (offset past replacement=w233:i32)  [unwired: 4 in, 3 out]
                      n117 = Less Than 0?(x=w233) -> (x < 0?=w234:bool)
                      n118 = case shown="False" w234 {
                        tunnel: [TRUE FALSE] -> w224
                        tunnel: w222 -> [w235 _]
                        frame False {
                          "End Number" <- w235
                        }
                        frame True {
                        }
                      }
                      n119 = Or(x=w224, y=w225) -> (x .or. y?=w223:bool)
                    }
                    n120 = Equal?(x=w159, y=w158) -> (x = y?=w145:bool)
                    n121 = Equal?(x=w165, y=w164) -> (x = y?=w143:bool)
                    n122 = Unbundle By Name "АУ2ГУИ_"(w163) -> ("Names"=w160:string[])
                    n123 = Unbundle By Name "АУ2ГУИ_"(w162) -> ("Names"=w161:string[])
                    n124 = Equal?(x=w160, y=w161) -> (x = y?=w144:bool)
                    n125 = Compound Arithmetic op=AND(w141, w140, w139, w147, w146, w145, w144, w143) -> (w142:bool)
                    n126 = case shown="True" w142 {
                      tunnel: w147 -> [w221 _]
                      tunnel: w146 -> [w220 _]
                      tunnel: w145 -> [w219 _]
                      tunnel: w144 -> [w218 _]
                      tunnel: w143 -> [w217 _]
                      tunnel: w141 -> [w204 _]
                      tunnel: w140 -> [w202 _]
                      tunnel: w139 -> [w201 _]
                      frame False {
                        n127 = Build Array(w204, w202, w201, w221, w220, w219, w218, w217) -> (w211:bool[])
                        n128 = Search 1D Array(1D array=w211, element=FALSE) -> (index of element=w208:i32)  [unwired: 1 in]
                        n129 = Build Array("Входные порты АУ и  выходные порты ВОУ", "Выходные порты АУ и  входные порты ВОУ", "Порты АУ, ВОУ и БВ", "БУС2ВОУ_", "БВ2БУС_", "БУС2БВ_", "АУ2ГУИ_", "КОМ2АУ_") -> (w209:string[])
                        n130 = Index Array(array=w209, index=w208) -> (element=w206:string)
                        n131 = Concatenate Strings("Ошибка загрузки алгоблоков! \nПроверьте соответствие следующих входных данных: " ("message"), w206) -> (w205:string)
                        n132 = One Button Dialog(message=w205) -> ()  [unwired: 1 in, 1 out]
                      }
                      frame True {
                      }
                    }
                  }
                }
              }
              frame #1 {
                n133 = case shown="True" w238 {
                  selector: w238 -> [_ w241]
                  frame False {
                  }
                  frame True {
                    n134 = flat-sequence {
                      tunnel: w241 -> [w245]
                      frame #0 {
                        n135 = local read "Проект"() -> (w243:path)
                        n136 = Path To String(path=w243) -> (string=w242:string)
                        n137 = dll-call lib="C:/Users/cald9/OneDrive/Документы/GitHub/MyComplex/DLL-s/MakeFullImmitationStepDLL/Release/MakeFullImmitationStepDLL.dll" fn="?loadNewDlls@@YAHPAPAULabViewString@@@Z" label="Load NEW DLLs"("path"=w242) -> ("error"=→"error":i32)  [unwired: 4 in, 2 out]
                      }
                      frame #1 {
                        w248 = T8."Enabled" ("Disabled")
                        n138 = local write "Верификация запущена"(w245) -> ()
                        n139 = local write "Pause"(FALSE ("Pause")) -> ()
                        n140 = property on="Pause" class="Bool (strict)"("DisabledEnum"=w248) -> ()  [unwired: 2 in, 2 out]
                        n141 = property on="Stop Ver Button" class="Bool (strict)"("DisabledEnum"=w248) -> ()  [unwired: 2 in, 2 out]
                        n142 = property on="START Button" class="Bool (strict)"("DisabledEnum"=T8."Disabled and Grayed Out" ("Disabled")) -> ()  [unwired: 2 in, 2 out]
                      }
                    }
                  }
                }
                n143 = Send Notification(notification=enum16{"no command", "refresh"}."refresh", notifier=w240) -> ()  [unwired: 1 in, 2 out]
              }
            }
          }
        }
      }
      event "Pause": Mouse Down {
        n144 = event-data() -> ()  [unwired: 1 in, 7 out]
        n145 = local read "Верификация запущена"() -> (w250:bool)
        n146 = Not(x=w250) -> (.not. x?=w249:bool)
        n147 = local write "Верификация запущена"(w249) -> ()
      }
      event "Stop Ver Button": Mouse Down {
        n148 = event-data() -> ()  [unwired: 1 in, 7 out]
        n149 = flat-sequence {
          frame #0 {
            n150 = dll-call lib="C:/Users/cald9/OneDrive/Документы/GitHub/MyComplex/DLL-s/MakeFullImmitationStepDLL/Release/MakeFullImmitationStepDLL.dll" fn="?freeAllDlls@@YAXXZ" label="FREE DLLs"() -> ()  [unwired: 4 in, 2 out]
          }
          frame #1 {
            w252 = T8."Disabled and Grayed Out" ("Disabled")
            n151 = local write "Pause"(FALSE ("Pause")) -> ()
            n152 = local write "Верификация запущена"(FALSE ("VerificationRunning")) -> ()
            n153 = property on="START Button" class="Bool (strict)"("DisabledEnum"=T8."Enabled" ("Disabled")) -> ()  [unwired: 2 in, 2 out]
            n154 = property on="Stop Ver Button" class="Bool (strict)"("DisabledEnum"=w252) -> ()  [unwired: 2 in, 2 out]
            n155 = property on="Pause" class="Bool (strict)"("DisabledEnum"=w252) -> ()  [unwired: 2 in, 2 out]
          }
        }
      }
      event Menu Selection (User) {
        n156 = event-data() -> ("MenuRef"=w256:refnum<k9>, "ItemTag"=w257:string)  [unwired: 1 in, 4 out]
        n157 = case shown="\"LoadIMG\"" w257 {
          tunnel: w256 -> [w259 w305 w306 w347 w351 w353]
          tunnel: [w259 w305 w306 w347 w351 w353] -> w255
          frame "New" {
            n158 = local read "Проект"() -> (w260:path)
            n159 = call "File Dialog2"("start path"=w260, "prompt"="Выберите папку, в которой хотите создать проект" ("default name"), "button label"="Создать проект в текущей папке" ("pattern label"), "default name"="Progect") -> ("selected path"=w263:path, "exists"=w262:bool, "cancelled"=w261:bool)  [unwired: 8 in, 1 out]
            "selected path" <- w263
            n160 = case shown="False" w261 {
              tunnel: w263 -> [w268 _]
              tunnel: w262 -> [w267 _]
              frame False {
                n161 = case shown="True" w267 {
                  tunnel: w268 -> [_ w269]
                  frame False {
                  }
                  frame True {
                    n162 = call "CreateNewProgect.vi"("selected path"=w269) -> ("Boolean"=w270:bool)
                    n163 = case shown="True" w270 {
                      selector: w270 -> [_ w303]
                      tunnel: w269 -> [_ w278]
                      frame False {
                      }
                      frame True {
                        w273 = T8."Disabled and Grayed Out" ("Disabled")
                        w283 = "Section 1" ("section")
                        w285 = path ""
                        n164 = Current VI's Menubar() -> (w275:refnum<k9>)
                        n165 = local write "Pause"(FALSE ("Pause")) -> ()
                        n166 = local write "Верификация запущена"(FALSE ("VerificationRunning")) -> ()
                        n167 = Strip Path(path=w278) -> (name=w279:string)  [unwired: 1 out]
                        n168 = local write "Project"(w279) -> ()
                        n169 = Set Menu Item Info(7:"LoadIMG" ("item tag"), 9:TRUE ("enabled"), 11:w275) -> ()  [unwired: 4 in, 2 out]
                        n170 = local write "Scalar"(w303) -> ()
                        n171 = Build Path(base path=w278, name or relative path="progect_cfg.ini") -> (appended path=w294:path)
                        n172 = call <vilib>:"Application Directory.vi"() -> ("Application Directory"=w302:path)
                        n173 = local write "Проект"(w278) -> ()
                        n174 = call <vilib>:"Open Config Data.vi"("create file if necessary (T)"=TRUE, "configuration file path"=w294) -> ("error out"=w292:errorcluster, "refnum"=w291:T9)  [unwired: 7 in, 1 out]
                        n175 = Build Path(base path=w302, name or relative path="cfg.ini") -> (appended path=w300:path)
                        n176 = local read "subpanel VI ref"() -> (w281:refnum<vi>)
                        n177 = call <vilib>:"Open Config Data.vi"("configuration file path"=w300) -> ("refnum"=w299:T9)  [unwired: 8 in, 2 out]
                        n178 = call-poly <vilib>:"Write Key.vi"("section"=w283, "error in (no error)"=w292, "value"=w285, "key"="pic", "refnum"=w291) -> ("error out"=w288:errorcluster, "refnum out"=w289:T9)  [unwired: 4 in, 1 out]
                        n179 = Equal?(x=w281, y=refnum<k0> refnum) -> (x = y?=w280:bool)
                        n180 = call-poly <vilib>:"Write Key.vi"("section"="Section 1", "value"=w278, "key"="Progect", "refnum"=w299) -> ("refnum out"=w296:T9)  [unwired: 5 in, 2 out]
                        n181 = case shown="False" w280 {
                          tunnel: w281 -> [w304 _]
                          frame False {
                            n182 = invoke on="Sub Panel" class="SubPnl" method="Remove VI"() -> ()  [unwired: 3 in, 3 out]
                            n183 = Close Reference(reference=w304) -> ()  [unwired: 1 in, 1 out]
                          }
                          frame True {
                          }
                        }
                        n184 = call-poly <vilib>:"Write Key.vi"("section"=w283, "error in (no error)"=w288, "value"=w285, "key"="xml", "refnum"=w289) -> ("error out"=w286:errorcluster, "refnum out"=w287:T9)  [unwired: 4 in, 1 out]
                        n185 = call <vilib>:"Close Config Data.vi"("refnum"=w296) -> ()  [unwired: 9 in, 2 out]
                        n186 = call <vilib>:"Close Config Data.vi"("error in (no error)"=w286, "refnum"=w287) -> ()  [unwired: 8 in, 2 out]
                        n187 = property on="START Button" class="Bool (strict)"("DisabledEnum"=T8."Enabled" ("Disabled")) -> ()  [unwired: 2 in, 2 out]
                        n188 = property on="Stop Ver Button" class="Bool (strict)"("DisabledEnum"=w273) -> ()  [unwired: 2 in, 2 out]
                        n189 = property on="Pause" class="Bool (strict)"("DisabledEnum"=w273) -> ()  [unwired: 2 in, 2 out]
                      }
                    }
                  }
                }
                "exists" <- w267
              }
              frame True {
              }
            }
          }
          frame Default {
          }
          frame "LoadIMG" {
            n190 = flat-sequence {
              frame #0 {
                n191 = local read "Проект"() -> (w307:path)
                n192 = call "File Dialog3"("start path"=w307, "prompt"="Выберите файл изображения", "pattern (all files)"="*.jpg; *.bmp; *.png") -> ("selected path"=w309:path, "cancelled"=w308:bool)  [unwired: 9 in, 2 out]
                n193 = case shown="False" w308 {
                  tunnel: w309 -> [w314 _]
                  tunnel: w307 -> [w312 _]
                  frame False {
                    n194 = call "File Dialog4"("start path"=w312, "prompt"="Выберите файл XML", "pattern (all files)"="*.xml") -> ("selected path"=w317:path, "cancelled"=w313:bool)  [unwired: 9 in, 2 out]
                    n195 = case shown="False" w313 {
                      tunnel: w317 -> [w319 _]
                      tunnel: w314 -> [w318 _]
                      frame False {
                        n196 = local read "Проект"() -> (w320:path)
                        n197 = flat-sequence {
                          tunnel: w320 -> [w324]
                          tunnel: w319 -> [w323]
                          tunnel: w318 -> [w322]
                          tunnel: w320 -> [w342]
                          frame #0 {
                            w333 = "Section 1" ("section")
                            n198 = Build Path(base path=w324, name or relative path="progect_cfg.ini") -> (appended path=w325:path)
                            n199 = call <vilib>:"Open Config Data.vi"("create file if necessary (T)"=TRUE, "configuration file path"=w325) -> ("error out"=w327:errorcluster, "refnum"=w328:T9)  [unwired: 7 in, 1 out]
                            n200 = call-poly <vilib>:"Write Key.vi"("section"=w333, "error in (no error)"=w327, "value"=w322, "key"="pic", "refnum"=w328) -> ("error out"=w332:errorcluster, "refnum out"=w335:T9)  [unwired: 4 in, 1 out]
                            n201 = call-poly <vilib>:"Write Key.vi"("section"=w333, "error in (no error)"=w332, "value"=w323, "key"="xml", "refnum"=w335) -> ("error out"=w330:errorcluster, "refnum out"=w334:T9)  [unwired: 4 in, 1 out]
                            n202 = call <vilib>:"Close Config Data.vi"("error in (no error)"=w330, "refnum"=w334) -> ()  [unwired: 8 in, 2 out]
                          }
                          frame #1 {
                            n203 = local read "subpanel VI ref"() -> (w336:refnum<vi>)
                            n204 = Equal?(x=w336, y=refnum<k0> refnum) -> (x = y?=w337:bool)
                            n205 = case shown="False" w337 {
                              tunnel: w336 -> [w339 _]
                              frame False {
                                n206 = invoke on="Sub Panel" class="SubPnl" method="Remove VI"() -> (error out=w340:errorcluster)  [unwired: 3 in, 2 out]
                                n207 = Close Reference(reference=w339, error in (no error)=w340) -> ()  [unwired: 1 out]
                              }
                              frame True {
                              }
                            }
                          }
                          frame #2 {
                            n208 = control-ref of="algInputPorts"() -> ()  [unwired: 1 out]
                            n209 = control-ref of="algOutputPorts"() -> ()  [unwired: 1 out]
                            n210 = call "Load PIC and XML.vi"("selected path"=w342) -> ("toChanger"=w341:T1, "vi refnum"=w345:refnum<vi>)  [unwired: 2 in]
                            n211 = local write "toChanger"(w341) -> ()
                            n212 = Equal?(x=refnum<k0> refnum, y=w345) -> (x = y?=w344:bool)
                            n213 = case shown="False" w344 {
                              tunnel: w345 -> [w346 _]
                              frame False {
                                n214 = invoke on="Sub Panel" class="SubPnl" method="Insert VI"("VI Ref"=w346) -> ()  [unwired: 3 in, 4 out]
                              }
                              frame True {
                              }
                            }
                          }
                        }
                      }
                      frame True {
                      }
                    }
                  }
                  frame True {
                  }
                }
              }
            }
          }
          frame "ProjDescr" {
            n215 = local read "Проект"() -> (w348:path)
            n216 = call <vilib>:"System Exec.vi"("wait until completion? (T)"=FALSE, "working directory"=w348, "command line"="C:\\Program Files (x86)\\Notepad++\\notepad++.exe  \"Описание проекта.txt\"" ("name or relative path")) -> ()  [unwired: 5 in, 4 out]
          }
          frame "About" {
            n217 = One Button Dialog(message="Описание программы.\n\nКомплекс автоматической верификации промышленных алгоритмов управления.\n\nНачало работы:\n\n1)\tПроект -> Создать проект -> Создать проект в текущей директории. \nПосле этого в выбранной директории создадутся папки:\n- CA\n- VP \n- SCM\n- VM\nВ каждой папке появятся файлы-заготовки RCS с шаблоном кода на языке Reflex\n2)\tКнопка Редактирование открывает редактор с .rcs файлами.\n3)\tПосле редактирования кода на языке Reflex запускаем скрипт BUILD\n4)\tВывод скрипта делится на две части: Вывод транслятора из языка Reflex в язык C и вывод компилятора. \nВывод транслятора: Если пишется, что PASS ONE COMPLETE. PASS TWO COMPLETE. - Значит, ошибок в коде на языке Reflex нет.\nВывод компилятора - стандартный вывоз компилятора  GCC. Если ошибок нет и появляется строчка Скопировано файлов - 1, то ошибок при создании DLL нет. \n5)\tЕсли нет ошибок и DLL сгенерировано, можно приступать к верификации.\nВ окне \"Окно верификации\" Нажмите кнопку запуска верификации. Верификация началась.\nСостояние алгоблоков можно проверить, открыв панели состояний алгоблоков БУС, БУВ, ВОУ И АУ.\n\nПо завершению верификации появится сообщение \"Верификация завершена!\"\n\nТребуемые префиксы сообщений алгоблоков:\nАУ:\n- КОМ2АУ_ - входные сообщения алгоритма;\n- АУ2ГИО_ - выходные сообщения алгоритма;\nВОУ:\n- БУС2ВОУ_ - входные сообщения от блока управления сценариями имитатору объекта \n- ВОУ2ГИО_ - выходные сообщения от объекта управления\nБУС:\n- БУС2ВОУ_ - выходные команды объекту управления\n- КОМ2АУ_ - выходные сообщения алгоритму\n- БУС2БВ_ - выходные сообщения верификатору\n- БВ2БУС_ - входные сообщения от верификатора\nБВ:\n- АУ2ГИО__ - выходные сообщения алгоритма;\n- БУС2БВ_ - входные сообщения от БУС\n- БВ2БУС_ - выходные сообщения от для БВ\n- БВ2ГИО_ = выходные команды для ГИО\n  ") -> ()  [unwired: 1 in, 1 out]
          }
          frame "Open" {
            n218 = call <vilib>:"Application Directory.vi"() -> ("Application Directory"=w357:path)
            n219 = call "File Dialog"("start path"=w357, "prompt"="Выбрать файл проекта" ("default name"), "button label"="Выбрать проект" ("pattern label")) -> ("selected path"=w354:path, "cancelled"=w355:bool)  [unwired: 9 in, 2 out]
            n220 = case shown="False" w355 {
              tunnel: w354 -> [w359 _]
              frame False {
                n221 = List Folder(path=w359) -> (folder names=w369:string[])  [unwired: 3 in, 3 out]
                n222 = Search 1D Array(1D array=w369, element="VP") -> (index of element=w366:i32)  [unwired: 1 in]
                n223 = Search 1D Array(1D array=w369, element="CA") -> (index of element=w367:i32)  [unwired: 1 in]
                n224 = Search 1D Array(1D array=w369, element="VM") -> (index of element=w364:i32)  [unwired: 1 in]
                n225 = Search 1D Array(1D array=w369, element="SCM") -> (index of element=w365:i32)  [unwired: 1 in]
                n226 = Build Array(w367, w366, w365, w364) -> (w363:i32[])
                n227 = call "Convert to Dynamic Data"("Array"=w363) -> ("Dynamic Data Type"=w362:dynamicdata)  [unwired: 3 in]
                n228 = call "Greater or Equal"("Constant Value to Compare Against"=0, "Operand 1"=w362) -> ("Result"=w361:dynamicdata)  [unwired: 8 in, 1 out]
                n229 = call "Convert from Dynamic Data"("Dynamic Data Type"=w361) -> ("Scalar"=w360:bool)  [unwired: 3 in]
                "Scalar" <- w360
                n230 = case shown="True" w360 {
                  tunnel: w359 -> [_ w379]
                  frame False {
                    n231 = One Button Dialog(message="Wrong progect path!") -> ()  [unwired: 1 in, 1 out]
                  }
                  frame True {
                    w377 = T8."Disabled and Grayed Out" ("Disabled")
                    n232 = flat-sequence {
                      tunnel: w379 -> [w396]
                      tunnel: [w396] -> w380
                      tunnel: w380 -> [w399]
                      frame #0 {
                        n233 = local read "subpanel VI ref"() -> (w393:refnum<vi>)
                        n234 = Equal?(x=w393, y=refnum<k0> refnum) -> (x = y?=w394:bool)
                        n235 = case shown="False" w394 {
                          tunnel: w393 -> [w397 _]
                          frame False {
                            n236 = invoke on="Sub Panel" class="SubPnl" method="Remove VI"() -> ()  [unwired: 3 in, 3 out]
                            n237 = Close Reference(reference=w397) -> ()  [unwired: 1 in, 1 out]
                          }
                          frame True {
                          }
                        }
                      }
                      frame #1 {
                        n238 = call "Load PIC and XML.vi"("selected path"=w399) -> ("toChanger"=w398:T1, "vi refnum"=w400:refnum<vi>)  [unwired: 2 in]
                        n239 = local write "toChanger"(w398) -> ()
                        n240 = Equal?(x=refnum<k0> refnum, y=w400) -> (x = y?=w401:bool)
                        n241 = case shown="False" w401 {
                          tunnel: w400 -> [w403 _]
                          frame False {
                            n242 = invoke on="Sub Panel" class="SubPnl" method="Insert VI"("VI Ref"=w403) -> ()  [unwired: 3 in, 4 out]
                          }
                          frame True {
                          }
                        }
                      }
                    }
                    n243 = property on="START Button" class="Bool (strict)"("DisabledEnum"=T8."Enabled" ("Disabled")) -> ()  [unwired: 2 in, 2 out]
                    n244 = local write "Pause"(FALSE ("Pause")) -> ()
                    n245 = local write "Верификация запущена"(FALSE ("VerificationRunning")) -> ()
                    n246 = property on="Stop Ver Button" class="Bool (strict)"("DisabledEnum"=w377) -> ()  [unwired: 2 in, 2 out]
                    n247 = property on="Pause" class="Bool (strict)"("DisabledEnum"=w377) -> ()  [unwired: 2 in, 2 out]
                    n248 = local write "Проект"(w379) -> ()
                    n249 = Strip Path(path=w379) -> (name=w392:string)  [unwired: 1 out]
                    n250 = local read "Проект"() -> (w384:path)
                    n251 = call <vilib>:"Application Directory.vi"() -> ("Application Directory"=w391:path)
                    n252 = Current VI's Menubar() -> (w383:refnum<k9>)
                    n253 = local write "Project"(w392) -> ()
                    n254 = Build Path(base path=w391, name or relative path="cfg.ini") -> (appended path=w389:path)
                    n255 = call <vilib>:"Open Config Data.vi"("configuration file path"=w389) -> ("refnum"=w388:T9)  [unwired: 8 in, 2 out]
                    n256 = call-poly <vilib>:"Write Key.vi"("section"="Section 1", "value"=w384, "key"="Progect", "refnum"=w388) -> ("refnum out"=w386:T9)  [unwired: 5 in, 2 out]
                    n257 = Set Menu Item Info(7:"LoadIMG" ("item tag"), 9:TRUE ("enabled"), 11:w383) -> ()  [unwired: 4 in, 2 out]
                    n258 = call <vilib>:"Close Config Data.vi"("refnum"=w386) -> ()  [unwired: 9 in, 2 out]
                  }
                }
              }
              frame True {
              }
            }
          }
        }
        n259 = Enable Menu Tracking(3:TRUE ("enable (T)"), 4:w255) -> ()  [unwired: 1 in, 2 out]
      }
      event "Открыть панель АУ": Mouse Up {
        n260 = event-data() -> ()  [unwired: 1 in, 7 out]
        n261 = local read "CA vi reference"() -> (w446:refnum<vi>)
        n262 = invoke class="VI" method="FP.Open"(reference=w446) -> (reference out=w445:refnum<vi>, error out=w443:errorcluster)  [unwired: 4 in, 3 out]
        n263 = control-ref of="CA DESCR"() -> (w442:refnum<vi>)
        n264 = invoke class="VI" method="Ctrl Val.Set"(reference=w445, error in=w443, "Control Name"="PORTS", "Value"=w442) -> (reference out=w441:refnum<vi>, error out=w440:errorcluster)  [unwired: 1 in, 3 out]
        n265 = control-ref of="algInputPorts"() -> (w438:refnum<vi>)
        n266 = invoke class="VI" method="Ctrl Val.Set"(reference=w441, error in=w440, "Control Name"="INP", "Value"=w438) -> (reference out=w436:refnum<vi>, error out=w435:errorcluster)  [unwired: 1 in, 3 out]
        n267 = control-ref of="algOutputPorts"() -> (w434:refnum<vi>)
        n268 = invoke class="VI" method="Ctrl Val.Set"(reference=w436, error in=w435, "Control Name"="OUTP", "Value"=w434) -> (reference out=w431:refnum<vi>, error out=w430:errorcluster)  [unwired: 1 in, 3 out]
        n269 = control-ref of="CA PROCESSES"() -> (w424:refnum<vi>)
        n270 = invoke class="VI" method="Ctrl Val.Set"(reference=w431, error in=w430, "Control Name"="Processes", "Value"=w424) -> (reference out=w429:refnum<vi>, error out=w428:errorcluster)  [unwired: 1 in, 3 out]
        n271 = control-ref of="CA STATES"() -> (w423:refnum<vi>)
        n272 = invoke class="VI" method="Ctrl Val.Set"(reference=w429, error in=w428, "Control Name"="States", "Value"=w423) -> (reference out=w426:refnum<vi>, error out=w425:errorcluster)  [unwired: 1 in, 3 out]
        n273 = control-ref of="algStates"() -> (w422:refnum<vi>)
        n274 = invoke class="VI" method="Ctrl Val.Set"(reference=w426, error in=w425, "Control Name"="AlgStates", "Value"=w422) -> (reference out=w421:refnum<vi>, error out=w420:errorcluster)  [unwired: 1 in, 3 out]
        n275 = control-ref of="CA2GUI Msg Cluster Array"() -> (w404:refnum<vi>)
        n276 = invoke class="VI" method="Ctrl Val.Set"(reference=w421, error in=w420, "Control Name"="CA2GUI", "Value"=w404) -> (reference out=w418:refnum<vi>, error out=w417:errorcluster)  [unwired: 1 in, 3 out]
        n277 = control-ref of="algOutputMsgs"() -> (w416:refnum<vi>)
        n278 = invoke class="VI" method="Ctrl Val.Set"(reference=w418, error in=w417, "Control Name"="algOutputMsgs", "Value"=w416) -> (reference out=w413:refnum<vi>, error out=w412:errorcluster)  [unwired: 1 in, 3 out]
        n279 = control-ref of="CA input vars"() -> (w411:refnum<vi>)
        n280 = invoke class="VI" method="Ctrl Val.Set"(reference=w413, error in=w412, "Control Name"="INPUT VARS", "Value"=w411) -> (reference out=w410:refnum<vi>, error out=w409:errorcluster)  [unwired: 1 in, 3 out]
        n281 = control-ref of="CA output vars"() -> (w405:refnum<vi>)
        n282 = invoke class="VI" method="Ctrl Val.Set"(reference=w410, error in=w409, "Control Name"="OUTPUT VARS", "Value"=w405) -> (reference out=w408:refnum<vi>, error out=w407:errorcluster)  [unwired: 1 in, 3 out]
        n283 = invoke class="VI" method="Run VI"(reference=w408, error in=w407, "Wait until done"=FALSE ("Wait Until Done")) -> (error out=→"error out":errorcluster)  [unwired: 2 in, 4 out]
      }
      event "Открыть панель ВОУ": Mouse Up {
        n284 = event-data() -> ()  [unwired: 1 in, 7 out]
        n285 = local read "VP vi reference"() -> (w490:refnum<vi>)
        n286 = invoke class="VI" method="FP.Open"(reference=w490) -> (reference out=w462:refnum<vi>)  [unwired: 4 in, 4 out]
        n287 = control-ref of="VP Cluster"() -> (w453:refnum<vi>)
        n288 = invoke class="VI" method="Ctrl Val.Set"(reference=w462, "Control Name"="PORTS", "Value"=w453) -> (reference out=w488:refnum<vi>, error out=w487:errorcluster)  [unwired: 2 in, 3 out]
        n289 = control-ref of="algOutputPorts"() -> (w460:refnum<vi>)
        n290 = invoke class="VI" method="Ctrl Val.Set"(reference=w488, error in=w487, "Control Name"="INP", "Value"=w460) -> (reference out=w484:refnum<vi>, error out=w483:errorcluster)  [unwired: 1 in, 3 out]
        n291 = control-ref of="algInputPorts"() -> (w459:refnum<vi>)
        n292 = invoke class="VI" method="Ctrl Val.Set"(reference=w484, error in=w483, "Control Name"="OUTP", "Value"=w459) -> (reference out=w480:refnum<vi>, error out=w479:errorcluster)  [unwired: 1 in, 3 out]
        n293 = control-ref of="VP PROCESSES"() -> (w458:refnum<vi>)
        n294 = invoke class="VI" method="Ctrl Val.Set"(reference=w480, error in=w479, "Control Name"="Processes", "Value"=w458) -> (reference out=w478:refnum<vi>, error out=w477:errorcluster)  [unwired: 1 in, 3 out]
        n295 = control-ref of="VP STATES"() -> (w457:refnum<vi>)
        n296 = invoke class="VI" method="Ctrl Val.Set"(reference=w478, error in=w477, "Control Name"="States", "Value"=w457) -> (reference out=w475:refnum<vi>, error out=w474:errorcluster)  [unwired: 1 in, 3 out]
        n297 = control-ref of="vplantStates"() -> (w456:refnum<vi>)
        n298 = invoke class="VI" method="Ctrl Val.Set"(reference=w475, error in=w474, "Control Name"="VPStates", "Value"=w456) -> (reference out=w473:refnum<vi>, error out=w472:errorcluster)  [unwired: 1 in, 3 out]
        n299 = control-ref of="VP 2 GUI Msg Cluster Array"() -> (w452:refnum<vi>)
        n300 = invoke class="VI" method="Ctrl Val.Set"(reference=w473, error in=w472, "Control Name"="VP2GUI", "Value"=w452) -> (reference out=w470:refnum<vi>, error out=w469:errorcluster)  [unwired: 1 in, 3 out]
        n301 = control-ref of="virtualPlant2GUIOutputMsgs"() -> (w450:refnum<vi>)
        n302 = invoke class="VI" method="Ctrl Val.Set"(reference=w470, error in=w469, "Control Name"="VPOutputMsgs", "Value"=w450) -> (reference out=w467:refnum<vi>, error out=w466:errorcluster)  [unwired: 1 in, 3 out]
        n303 = control-ref of="VP input vars"() -> (w455:refnum<vi>)
        n304 = invoke class="VI" method="Ctrl Val.Set"(reference=w467, error in=w466, "Control Name"="INPUT VARS", "Value"=w455) -> (reference out=w465:refnum<vi>, error out=w464:errorcluster)  [unwired: 1 in, 3 out]
        n305 = control-ref of="VP output vars"() -> (w454:refnum<vi>)
        n306 = invoke class="VI" method="Ctrl Val.Set"(reference=w465, error in=w464, "Control Name"="OUTPUT VARS", "Value"=w454) -> (reference out=w461:refnum<vi>)  [unwired: 1 in, 4 out]
        n307 = invoke class="VI" method="Run VI"(reference=w461, "Wait until done"=FALSE ("Wait Until Done")) -> (error out=w449:errorcluster)  [unwired: 3 in, 4 out]
        n308 = local write "error out"(w449) -> ()
      }
      event "Открыть панель БУС": Mouse Up {
        n309 = event-data() -> ()  [unwired: 1 in, 7 out]
        n310 = local read "SCB vi reference"() -> (w531:refnum<vi>)
        n311 = invoke class="VI" method="FP.Open"(reference=w531) -> (reference out=w521:refnum<vi>, error out=w522:errorcluster)  [unwired: 4 in, 3 out]
        n312 = control-ref of="SCM PROCESSES"() -> (w500:refnum<vi>)
        n313 = invoke class="VI" method="Ctrl Val.Set"(reference=w521, error in=w522, "Control Name"="Processes", "Value"=w500) -> (reference out=w527:refnum<vi>, error out=w526:errorcluster)  [unwired: 1 in, 3 out]
        n314 = control-ref of="SCM STATES"() -> (w499:refnum<vi>)
        n315 = invoke class="VI" method="Ctrl Val.Set"(reference=w527, error in=w526, "Control Name"="States", "Value"=w499) -> (reference out=w524:refnum<vi>, error out=w523:errorcluster)  [unwired: 1 in, 3 out]
        n316 = control-ref of="scenarioStates"() -> (w498:refnum<vi>)
        n317 = invoke class="VI" method="Ctrl Val.Set"(reference=w524, error in=w523, "Control Name"="SCBStates", "Value"=w498) -> (reference out=w516:refnum<vi>, error out=w515:errorcluster)  [unwired: 1 in, 3 out]
        n318 = control-ref of="SCM2VM Msg Cluster Array"() -> (w497:refnum<vi>)
        n319 = invoke class="VI" method="Ctrl Val.Set"(reference=w516, error in=w515, "Control Name"="SCM2VM", "Value"=w497) -> (reference out=w518:refnum<vi>, error out=w517:errorcluster)  [unwired: 1 in, 3 out]
        n320 = control-ref of="scenarios2VerifierOutputMsgs"() -> (w493:refnum<vi>)
        n321 = invoke class="VI" method="Ctrl Val.Set"(reference=w518, error in=w517, "Control Name"="VMInputMsgs", "Value"=w493) -> (reference out=w510:refnum<vi>, error out=w509:errorcluster)  [unwired: 1 in, 3 out]
        n322 = control-ref of="SCM-SCM2VP Msg Cluster Array"() -> (w496:refnum<vi>)
        n323 = invoke class="VI" method="Ctrl Val.Set"(reference=w510, error in=w509, "Control Name"="SCM2VP", "Value"=w496) -> (reference out=w512:refnum<vi>, error out=w511:errorcluster)  [unwired: 1 in, 3 out]
        n324 = control-ref of="scenarios2VirtPlantOutputMsgs"() -> (w492:refnum<vi>)
        n325 = invoke class="VI" method="Ctrl Val.Set"(reference=w512, error in=w511, "Control Name"="VPInputMsgs", "Value"=w492) -> (reference out=w504:refnum<vi>, error out=w503:errorcluster)  [unwired: 1 in, 3 out]
        n326 = control-ref of="SCM2CA Msg Cluster Array"() -> (w495:refnum<vi>)
        n327 = invoke class="VI" method="Ctrl Val.Set"(reference=w504, error in=w503, "Control Name"="SCM2CA", "Value"=w495) -> (reference out=w506:refnum<vi>, error out=w505:errorcluster)  [unwired: 1 in, 3 out]
        n328 = control-ref of="scenarios2AlgOutputMsgs"() -> (w494:refnum<vi>)
        n329 = invoke class="VI" method="Ctrl Val.Set"(reference=w506, error in=w505, "Control Name"="СAInputMsgs", "Value"=w494) -> (reference out=w502:refnum<vi>, error out=w501:errorcluster)  [unwired: 1 in, 3 out]
        n330 = invoke class="VI" method="Run VI"(reference=w502, error in=w501, "Wait until done"=FALSE ("Wait Until Done")) -> (error out=w530:errorcluster)  [unwired: 2 in, 4 out]
        n331 = local write "error out"(w530) -> ()
      }
      event "Открыть панель БВ": Mouse Up {
        n332 = event-data() -> ()  [unwired: 1 in, 7 out]
        n333 = local read "VM vi reference"() -> (w587:refnum<vi>)
        n334 = invoke class="VI" method="FP.Open"(reference=w587) -> (reference out=w579:refnum<vi>)  [unwired: 4 in, 4 out]
        n335 = control-ref of="VM PROCESSES"() -> (w577:refnum<vi>)
        n336 = invoke class="VI" method="Ctrl Val.Set"(reference=w579, "Control Name"="Processes", "Value"=w577) -> (reference out=w584:refnum<vi>, error out=w583:errorcluster)  [unwired: 2 in, 3 out]
        n337 = control-ref of="VM STATES"() -> (w576:refnum<vi>)
        n338 = invoke class="VI" method="Ctrl Val.Set"(reference=w584, error in=w583, "Control Name"="States", "Value"=w576) -> (reference out=w581:refnum<vi>, error out=w580:errorcluster)  [unwired: 1 in, 3 out]
        n339 = control-ref of="verStates"() -> (w578:refnum<vi>)
        n340 = invoke class="VI" method="Ctrl Val.Set"(reference=w581, error in=w580, "Control Name"="VMStates", "Value"=w578) -> (reference out=w571:refnum<vi>, error out=w570:errorcluster)  [unwired: 1 in, 3 out]
        n341 = control-ref of="VM DESCR"() -> (w566:refnum<vi>)
        n342 = invoke class="VI" method="Ctrl Val.Set"(reference=w571, error in=w570, "Control Name"="PORTS", "Value"=w566) -> (reference out=w574:refnum<vi>, error out=w573:errorcluster)  [unwired: 1 in, 3 out]
        n343 = control-ref of="algInputPorts"() -> (w565:refnum<vi>)
        n344 = invoke class="VI" method="Ctrl Val.Set"(reference=w574, error in=w573, "Control Name"="INP", "Value"=w565) -> (reference out=w568:refnum<vi>, error out=w567:errorcluster)  [unwired: 1 in, 3 out]
        n345 = control-ref of="algOutputPorts"() -> (w564:refnum<vi>)
        n346 = invoke class="VI" method="Ctrl Val.Set"(reference=w568, error in=w567, "Control Name"="OUTP", "Value"=w564) -> (reference out=w562:refnum<vi>, error out=w561:errorcluster)  [unwired: 1 in, 3 out]
        n347 = control-ref of="VM input vars"() -> (w560:refnum<vi>)
        n348 = invoke class="VI" method="Ctrl Val.Set"(reference=w562, error in=w561, "Control Name"="INPUT VARS", "Value"=w560) -> (reference out=w549:refnum<vi>, error out=w548:errorcluster)  [unwired: 1 in, 3 out]
        n349 = control-ref of="CA2GUI Msg Cluster Array"() -> (w546:refnum<vi>)
        n350 = invoke class="VI" method="Ctrl Val.Set"(reference=w549, error in=w548, "Control Name"="CA2GUI", "Value"=w546) -> (reference out=w551:refnum<vi>, error out=w552:errorcluster)  [unwired: 1 in, 3 out]
        n351 = control-ref of="algOutputMsgs"() -> (w547:refnum<vi>)
        n352 = invoke class="VI" method="Ctrl Val.Set"(reference=w551, error in=w552, "Control Name"="algOutputMsgs", "Value"=w547) -> (reference out=w555:refnum<vi>, error out=w556:errorcluster)  [unwired: 1 in, 3 out]
        n353 = control-ref of="VM2GUI Msg Cluster Array"() -> (w545:refnum<vi>)
        n354 = invoke class="VI" method="Ctrl Val.Set"(reference=w555, error in=w556, "Control Name"="VM2GUI", "Value"=w545) -> (reference out=w558:refnum<vi>, error out=w559:errorcluster)  [unwired: 1 in, 3 out]
        n355 = control-ref of="verifier2GUIOutputMsgs"() -> (w544:refnum<vi>)
        n356 = invoke class="VI" method="Ctrl Val.Set"(reference=w558, error in=w559, "Control Name"="verifier2GUIOutputMsgs", "Value"=w544) -> (reference out=w540:refnum<vi>, error out=w539:errorcluster)  [unwired: 1 in, 3 out]
        n357 = control-ref of="VM2SCM Msg Cluster Array"() -> (w538:refnum<vi>)
        n358 = invoke class="VI" method="Ctrl Val.Set"(reference=w540, error in=w539, "Control Name"="VM2SCM", "Value"=w538) -> (reference out=w542:refnum<vi>, error out=w541:errorcluster)  [unwired: 1 in, 3 out]
        n359 = control-ref of="verifier2scenariousControlOutMsgs"() -> (w536:refnum<vi>)
        n360 = invoke class="VI" method="Ctrl Val.Set"(reference=w542, error in=w541, "Control Name"="verifier2scenariousControlOutMsgs", "Value"=w536) -> (reference out=w535:refnum<vi>, error out=w534:errorcluster)  [unwired: 1 in, 3 out]
        n361 = invoke class="VI" method="Run VI"(reference=w535, error in=w534, "Wait until done"=FALSE ("Wait Until Done")) -> (error out=w533:errorcluster)  [unwired: 2 in, 4 out]
        n362 = local write "error out"(w533) -> ()
      }
      event "stop": Mouse Down {
        n363 = event-data() -> ()  [unwired: 1 in, 7 out]
        n364 = Open Application Reference() -> (3:w589:refnum<vi>)  [unwired: 4 in, 1 out]
        n365 = property class="App"(reference=w589) -> (error out=w591:errorcluster, "App.AllVIs"=w590:string[])  [unwired: 1 in, 1 out]
        n366 = dll-call lib="C:/Users/cald9/OneDrive/Документы/GitHub/MyComplex/DLL-s/MakeFullImmitationStepDLL/Release/MakeFullImmitationStepDLL.dll" fn="?freeAllDlls@@YAXXZ" label="FREE DLLs"() -> ()  [unwired: 4 in, 2 out]
        n367 = for {
          tunnel: w590 -> [w594] mode=indexing
          tunnel: w591 -> [w599]
          n368 = Open VI Reference(vi path=w594, error in (no error)=w599) -> (vi reference=w598:refnum<vi>, error out=w597:errorcluster)  [unwired: 4 in]
          n369 = property class="VI"(reference=w598, error in=w597) -> (reference out=w595:refnum<vi>, "Front Panel.Open"=w596:bool)  [unwired: 1 out]
          n370 = case shown="False" w596 {
            tunnel: w595 -> [w600 w602]
            tunnel: [w600 w601] -> w593
            frame False {
            }
            frame True {
              n371 = invoke class="VI" method="FP.Close"(reference=w602) -> (reference out=w601:refnum<vi>)  [unwired: 2 in, 2 out]
            }
          }
          n372 = Close Reference(reference=w593) -> ()  [unwired: 1 in, 1 out]
        }
        n373 = flat-sequence {
          frame #0 {
            n374 = invoke on="Sub Panel" class="SubPnl" method="Remove VI"() -> ()  [unwired: 3 in, 3 out]
          }
          frame #1 {
            n375 = local read "subpanel VI ref"() -> (w592:refnum<vi>)
            n376 = Close Reference(reference=w592) -> ()  [unwired: 1 in, 1 out]
          }
        }
      }
      event Application Instance Close {
        n377 = event-data() -> ()  [unwired: 1 in, 3 out]
        n378 = dll-call lib="C:/Users/cald9/OneDrive/Документы/GitHub/MyComplex/DLL-s/MakeFullImmitationStepDLL/Release/MakeFullImmitationStepDLL.dll" fn="?freeAllDlls@@YAXXZ" label="FREE DLLs"() -> ()  [unwired: 4 in, 2 out]
      }
    }
    n379 = local read "Верификация запущена"() -> (→"Verification":bool)
    n380 = local read "Верификация запущена"() -> (w46:bool)
    n381 = case shown="True" w46 {
      tunnel: "Режим работы:" -> [_ w78]
      frame False {
      }
      frame True {
        n382 = Boolean To (0,1)(Boolean=w78) -> (0, 1=w77:i16)
        n383 = dll-call lib="C:/Users/cald9/OneDrive/Документы/GitHub/MyComplex/DLL-s/MakeFullImmitationStepDLL/Release/MakeFullImmitationStepDLL.dll" fn="?setMode@@YAXE@Z" label="setMode"("mode"=w77) -> (error out=w76:errorcluster)  [unwired: 5 in, 1 out]
        n384 = dll-call lib="C:/Users/cald9/OneDrive/Документы/GitHub/MyComplex/DLL-s/MakeFullImmitationStepDLL/Release/MakeFullImmitationStepDLL.dll" fn="?LLD@@YAHPAPAUPort@@0PAPAUArrayOfMessages@@111111PAPAUArrayOfStates@@222@Z" label="Init"(error in=w76, "algInputPorts"="algInputPorts", "algOutputPorts"="algOutputPorts", "scenarios2AlgOutputMsgs"="scenarios2AlgOutputMsgs", "scenarios2VirtPlantOutputMsgs"="scenarios2VirtPlantOutputMsgs", "scenarios2VerifierOutputMsgs"="scenarios2VerifierOutputMsgs", "verifier2scenariousControlOutMsgs,"="verifier2scenariousControlOutMsgs", "algOutputMsgs"="algOutputMsgs", "verifier2GUIOutputMsgs"="verifier2GUIOutputMsgs", "virtualPlant2GUIOutputMsgs"="virtualPlant2GUIOutputMsgs", "algStates"="algStates", "vplantStates"="vplantStates", "verStates"="verStates", "scenarioStates"="scenarioStates") -> ("algInputPorts"=w50:i8[], "algOutputPorts"=w49:i8[], "scenarios2AlgOutputMsgs"=w58:cluster{"MSG":i16, "param":i32, "Type":i16}[], "scenarios2VirtPlantOutputMsgs"=w56:cluster{"MSG":i16, "param":i32, "Type":i16}[], "scenarios2VerifierOutputMsgs"=w57:cluster{"MSG":i16, "param":i32, "Type":i16}[], "verifier2scenariousControlOutMsgs,"=w54:cluster{"MSG":i16, "param":i32, "Type":i16}[], "algOutputMsgs"=w61:T7, "verifier2GUIOutputMsgs"=w52:cluster{"MSG":i16, "param":i32, "Type":i16}[], "virtualPlant2GUIOutputMsgs"=w60:cluster{"MSG":i16, "param":i32, "Type":i16}[], "algStates"=w62:cluster{"TimeInState":u16, "cur_state":i8}[], "vplantStates"=w59:cluster{"TimeInState":u16, "cur_state":i8}[], "verStates"=w53:cluster{"TimeInState":u16, "cur_state":i8}[], "scenarioStates"=w55:cluster{"TimeInState":u16, "cur_state":i8}[])  [unwired: 3 in, 2 out]
        n385 = local write "scenarioStates"(w55) -> ()
        n386 = local write "verStates"(w53) -> ()
        n387 = local write "virtualPlant2GUIOutputMsgs"(w60) -> ()
        n388 = local write "verifier2GUIOutputMsgs"(w52) -> ()
        n389 = local write "algInputPorts"(w50) -> ()
        n390 = local write "algOutputPorts"(w49) -> ()
        n391 = local write "verifier2scenariousControlOutMsgs"(w54) -> ()
        n392 = local write "vplantStates"(w59) -> ()
        n393 = local write "algStates"(w62) -> ()
        n394 = local write "algOutputMsgs"(w61) -> ()
        n395 = local write "scenarios2VirtPlantOutputMsgs"(w56) -> ()
        n396 = local write "scenarios2VerifierOutputMsgs"(w57) -> ()
        n397 = local write "scenarios2AlgOutputMsgs"(w58) -> ()
        n398 = Array Size(array=w52) -> (size(s)=w51:i32)
        n399 = local read "toChanger"() -> (w48:T1)
        n400 = while {
          tunnel: w52 -> [w89] mode=indexing
          tunnel: w51 -> [w86]
          i -> [w87]
          stop <- w80 stop-if-true
          n401 = local read "End Number"() -> (w88:i32)
          n402 = Unbundle By Name(w89) -> ("MSG"=w85:i16)
          n403 = Equal?(x=w86, y=w87) -> (x = y?=w81:bool)
          n404 = Equal?(x=w85, y=i16 -1) -> (x = y?=w82:bool)
          n405 = Equal?(x=w85, y=w88) -> ()  [unwired: 1 out]
          n406 = case shown="False" FALSE {
            tunnel: [FALSE ("Верификация запущена") TRUE ("Верификация запущена")] -> w83
            frame False {
            }
            frame True {
              w91 = T8."Disabled and Grayed Out" ("Disabled")
              n407 = flat-sequence {
                frame #0 {
                  n408 = dll-call lib="C:/Users/cald9/OneDrive/Документы/GitHub/MyComplex/DLL-s/MakeFullImmitationStepDLL/Release/MakeFullImmitationStepDLL.dll" fn="?freeAllDlls@@YAXXZ" label="FREE DLLs"() -> ()  [unwired: 4 in, 2 out]
                  n409 = local write "Верификация запущена"(FALSE ("Верификация запущена")) -> ()
                }
                frame #1 {
                  n410 = One Button Dialog(message="Верификация завершена!") -> ()  [unwired: 1 in, 1 out]
                }
              }
              n411 = property on="START Button" class="Bool (strict)"("DisabledEnum"=T8."Enabled" ("Disabled")) -> ()  [unwired: 2 in, 2 out]
              n412 = property on="Stop Ver Button" class="Bool (strict)"("DisabledEnum"=w91) -> ()  [unwired: 2 in, 2 out]
              n413 = property on="Pause" class="Bool (strict)"("DisabledEnum"=w91) -> ()  [unwired: 2 in, 2 out]
            }
          }
          n414 = Compound Arithmetic op=OR(w83, w82, w81) -> (w80:bool)
        }
        n415 = call "Changer.vi"("toChanger"=w48, "out"=w49, "in"=w50) -> ()
      }
    }
    "Автоматический режим работы" <- "Режим работы:"
  }
  n416 = local write "Scalar"(TRUE ("Scalar")) -> ()
  "Project" <- "" ("Название проекта")
